vi "exampleloop.vi"() -> ()   [LabVIEW 2011]
uses:
  gumLV8p2/D/Labviewsoft/transport/GUMS/Kelvinox drivers/ITCAPPS - Copie.LLB/ITCSignal.ctl
  gumLV8p2/D/Labviewsoft/transport/GUMS/Kelvinox drivers/ITCAPPS - Copie.LLB/ITCSignals.ctl
  DAC/Visa name1.vi
  GlobalVar.vi
  stopButton.vi
  monochromatorcontrol/perHandlemonochromator.vi
  users/nicolas/PHySpec-SDK-1.0.0/Labview-example/libPhyspec/libPhyspec.lvlib
panel:
  out "Bloop gen":u32
  out "WVlenloop gen":u32
  out "Tloop gen":u32
  out "loopchange":u32
  out "DACindic":bool
  in  "Gain Cluster 2":T1={"Vsd"="Gate", "I 2probe 2"="Gate", "Vxy"="Gate", "Vxx"="Gate", "I leak BG"="Gate", "I leak TG"="Gate", "I Gain 1"=1000000.0, "V Gain 1"=1.0, "conversion factor BG"=1.0, "Vin / Vout 1"=1.0, "V Gain 2"=1.0, "Vin / Vout 2"=1.0, "V Gain 3"=1.0, "Vin / Vout 3"=1.0, "I Gain 2"=1000000.0, "I Gain 3"=1000000.0, "V BG"="Gate", "V TG"="Gate", "conversion factor TG"=1.0, "Vin / Vout 4"=1.0, "Vin / Vout 5"=1.0, "Manual Gain 1"=1.0, "Manual Gain 2"=1.0, "Manual Gain 3"=1.0} {"conversion factor TG" items=["1 V/V"=1.0, "4 V/V"=4.0, "15 V/V"=15.0, "30 V/V"=30.0, "45 V/V"=45.0]; "I Gain 3" items=["1"=1.0, "10"=10.0, "100"=100.0, "1K"=1000.0, "10K"=10000.0, "100K"=100000.0, "1M"=1000000.0, "10M"=10000000.0, "100M"=100000000.0, "1G"=1000000000.0]; "I Gain 2" items=["1"=1.0, "10"=10.0, "100"=100.0, "1K"=1000.0, "10K"=10000.0, "100K"=100000.0, "1M"=1000000.0, "10M"=10000000.0, "100M"=100000000.0, "1G"=1000000000.0]; "V Gain 3" items=["1"=1.0, "10"=10.0, "100"=100.0, "1K"=1000.0, "10K"=10000.0]; "V Gain 2" items=["1"=1.0, "10"=10.0, "100"=100.0, "1K"=1000.0, "10K"=10000.0]; "conversion factor BG" items=["1 V/V"=1.0, "4 V/V"=4.0, "15 V/V"=15.0, "30 V/V"=30.0, "45 V/V"=45.0]; "V Gain 1" items=["1"=1.0, "10"=10.0, "100"=100.0, "1K"=1000.0, "10K"=10000.0]; "I Gain 1" items=["1"=1.0, "10"=10.0, "100"=100.0, "1K"=1000.0, "10K"=10000.0, "100K"=100000.0, "1M"=1000000.0, "10M"=10000000.0, "100M"=100000000.0, "1G"=1000000000.0]}
  out "DAC 2 number":u8
  in  "EmptyAllArrays":bool
  in  "Sweep back to zero":bool
  out "counter":i32
  out "Num elements in col":i32[](array[numeric])
  out "Current col":i32
  in  "Refresh Rate [ms]":i32=1000 min=0
  out "Current sweep":dbl
  out "ITC ref":T2={"ITC"=0, "Signal"=enum."Sensor 3"}
  in  "Cancel run":bool
  out "DAC 1 number":u8
  out "DAC":refnum<visa-resource-name>
  out "K2400 2":refnum<visa-resource-name>
  out "Lockin1":refnum<visa-resource-name>
  out "K2400 1":refnum<visa-resource-name>
  out "Total sweep sequence":dbl[][](array[numeric])
  in  "Device Cluster":T4={"K2400 1"="", "K2400_1"=FALSE, "K2400 2"="", "K2400_2"=FALSE, "Lockin1"="", "Lockin1 present"=FALSE, "Lockin2"="", "Lockin2 present"=FALSE, "TIC"="", "Tcontrol"="OFF", "DMM1"="", "DMM1"=FALSE, "DMM2"="", "DMM2"=FALSE, "DAC"="", "DAC present"=FALSE, "DAC sweep"=0, "Bfield query"=FALSE, "Wvlen query"=FALSE, "ITC signal"={"ITC"=0, "Signal"=enum."Sensor 1"}, "DAC fix"=0}
  in  "Tab Control":T5(tab)
  in  "Sweep Toothsaw":bool
  in  "Loop Cluster":T6
  in  "START":bool
  in  "genTotalSequence":bool
  out "row state":i32[](array[numeric])
  out "Priority type array":string[](array[string])
  out "TotalPnts":dbl
  in  "Sweep back\nto zero?":bool
  in  "Conversion Factor Fix\n1 V = ??":dbl=1.0
  in  "Fix type":string(combo)
  in  "Sweep Bias":dbl[](array[numeric])
  in  "Fix Bias":dbl[](array[numeric])
  in  "Priority sweep":i32=2
  in  "Priority fix":i32=2
  in  "sweep start [V]":dbl=-1.0 min=-200.0 max=200.0
  in  "sweep stop [V]":dbl=-5.0 min=-250.0 max=250.0
  in  "Nb steps":i32=800
  in  "sweep stop 2 [V]":dbl min=-250.0 max=250.0
  in  "Nb steps 2":i32
  in  "Nb Sweep":i32=1
  in  "Nb steps fix2":i32
  in  "Fix stop 2":dbl min=-250.0 max=250.0
  in  "Nb steps fix":i32=800
  in  "Fix stop":dbl=-5.0 min=-250.0 max=250.0
  in  "Fix start":dbl=-1.0 min=-200.0 max=200.0
  in  "genSweepArray":bool
  in  "genFixArray":bool
  in  "Sweep Instrument":string(combo)
  in  "Conversion Factor Sweep\n1 V = ??":dbl=1.0
  in  "Fix Instrument":string(combo)
  in  "Sweep type":string(combo)
  in  "V step K2400 [V]":dbl=0.001
  in  "genSweepArray sweeploop":bool
  in  "genfixArray fixlooop simple":bool
  in  "T [K]":dbl[](array[numeric])
  in  "Priority T":i32=2
  in  "Nb T steps":i32=800
  in  "T stop [K]":dbl=-1.0 min=-200.0 max=200.0
  in  "T start [K]":dbl=-1.0 min=-200.0 max=200.0
  in  "genTarray":bool
  in  "Add T points":bool
  in  "Zero ramp Rate [T/min] 2":dbl=0.2 min=-200.0 max=200.0
  in  "Sweep Field back to zero":bool
  in  "B [T]":dbl[](array[numeric])
  in  "Priority B":i32=2
  in  "B start [T]":dbl=-1.0 min=-200.0 max=200.0
  in  "B stop [T]":dbl=-1.0 min=-200.0 max=200.0
  in  "Sweep Rate [T/min]":dbl=0.1 min=-200.0 max=200.0
  in  "Nb B steps":i32=800
  in  "GenBarray":bool
  in  "Add B points":bool
  in  "Set Persistent":bool=TRUE
  in  "Power stabilization":bool=TRUE
  in  "Wvlen Start [nm]":dbl=400.0
  in  "Wavelength [nm]":dbl[](array[numeric])
  in  "genWVLEN array":bool
  in  "Add wvlen points":bool
  in  "Nb Wvlen steps":i32=350
  in  "Wvlen stop [nm]":dbl=1100.0
  out "Laser Power [W]":dbl format="%#.2g"
  in  "File Basename":string
  out "Bias factor":dbl
  in  "SD bias [V]":dbl=-1.0 min=-200.0 max=200.0
  in  "Nb steps Increase 2":dbl=10.0
  in  "Gate Increase 2 (V)":dbl=0.1
  in  "Nb steps Increase":dbl=10.0
  in  "Gate Increase (V)":dbl=-0.1
  out "x .or. y?":bool
  in  "Step Delay (ms)":dbl=1000.0
  out "Total Progress":dbl(slide) scale=0.0..1.0
  in  "Nb Loop":i32
  out "Nb Loop Indicator":i32=2
  out "Nb Sweep Indicator":i32=3
  out "conversion factor sweep":dbl(ring)=1.0 items=["1 V/V"=1.0, "4 V/V"=4.0, "15 V/V"=15.0, "30 V/V"=30.0, "45 V/V"=45.0]
  in  "stop":bool
  in  "V step [V]":dbl=0.001
  in  "Folder Name":path=path "D:/users/marc/20180122_LiIon_EL/Freezing02/OutputHighT002p2.dat"
  # "Magnetic Field"
  # "Wavelength"
  # "IV Sweep Setting"
  # "IV Fix Setting"
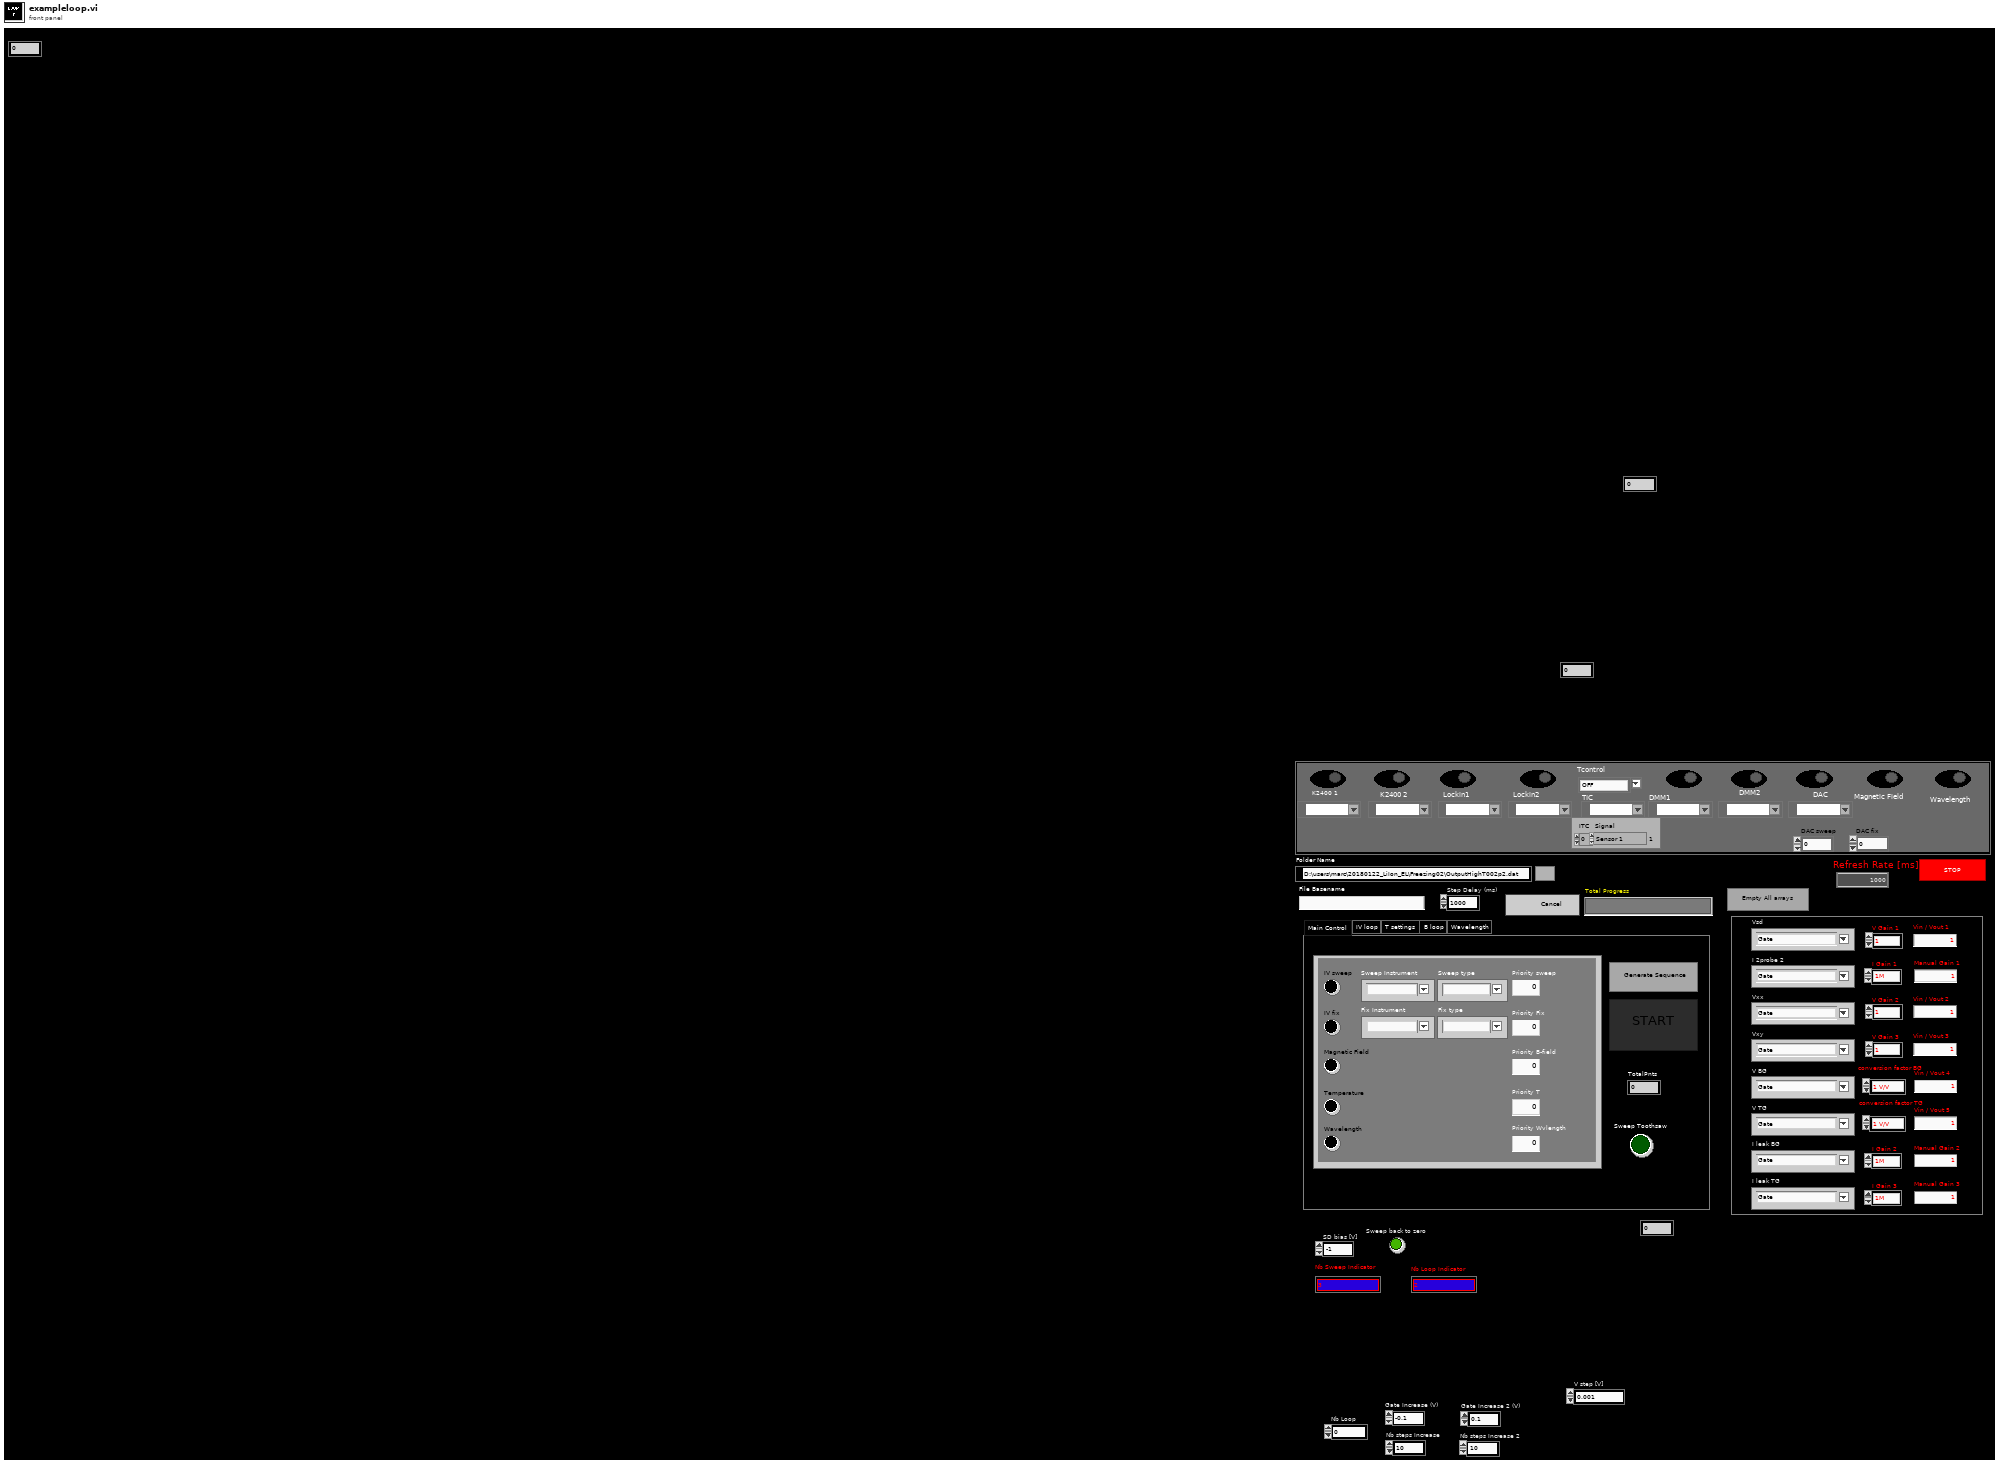
[diagram p1: front panel]
types:
  T1 = cluster{"Vsd":string, "I 2probe 2":string, "Vxy":string, "Vxx":string, "I leak BG":string, "I leak TG":string, "I Gain 1":dbl, "V Gain 1":dbl, "conversion factor BG":dbl, "Vin / Vout 1":dbl, "V Gain 2":dbl, "Vin / Vout 2":dbl, "V Gain 3":dbl, "Vin / Vout 3":dbl, "I Gain 2":dbl, "I Gain 3":dbl, "V BG":string, "V TG":string, "conversion factor TG":dbl, "Vin / Vout 4":dbl, "Vin / Vout 5":dbl, "Manual Gain 1":dbl, "Manual Gain 2":dbl, "Manual Gain 3":dbl}
  T2 = typedef "ITCSignal.ctl" = cluster{"ITC":u16, "Signal":T3}
  T3 = typedef "ITCSignals.ctl" = enum16{"Setpoint", "Sensor 1", "Sensor 2", "Sensor 3", "Needle Valve %", "Heater %"}
  T4 = cluster{"K2400 1":refnum<visa-resource-name>, "K2400_1":bool, "K2400 2":refnum<visa-resource-name>, "K2400_2":bool, "Lockin1":refnum<visa-resource-name>, "Lockin1 present":bool, "Lockin2":refnum<visa-resource-name>, "Lockin2 present":bool, "TIC":refnum<visa-resource-name>, "Tcontrol":string, "DMM1":refnum<visa-resource-name>, "DMM1":bool, "DMM2":refnum<visa-resource-name>, "DMM2":bool, "DAC":refnum<visa-resource-name>, "DAC present":bool, "DAC sweep":u8, "Bfield query":bool, "Wvlen query":bool, "ITC signal":T2, "DAC fix":u8}
  T5 = enum32{"Main Control", "IV loop", "T settings", "B loop", "Wavelength"}
  T6 = cluster{"Sweep Instrument":string, "Sweep type":string, "Fix Instrument":string, "Fix type":string, "IV sweep":bool, "IV fix":bool, "Magnetic Field":bool, "Temperature":bool, "Wavelength":bool, "Priority sweep":dbl, "Priority Fix":dbl, "Priority B-field":dbl, "Priority T":dbl, "Priority Wvlength":dbl}
  T7 = cluster{"Power Stabilization":bool, "Laser Power [W]":dbl, "Power precision":dbl}
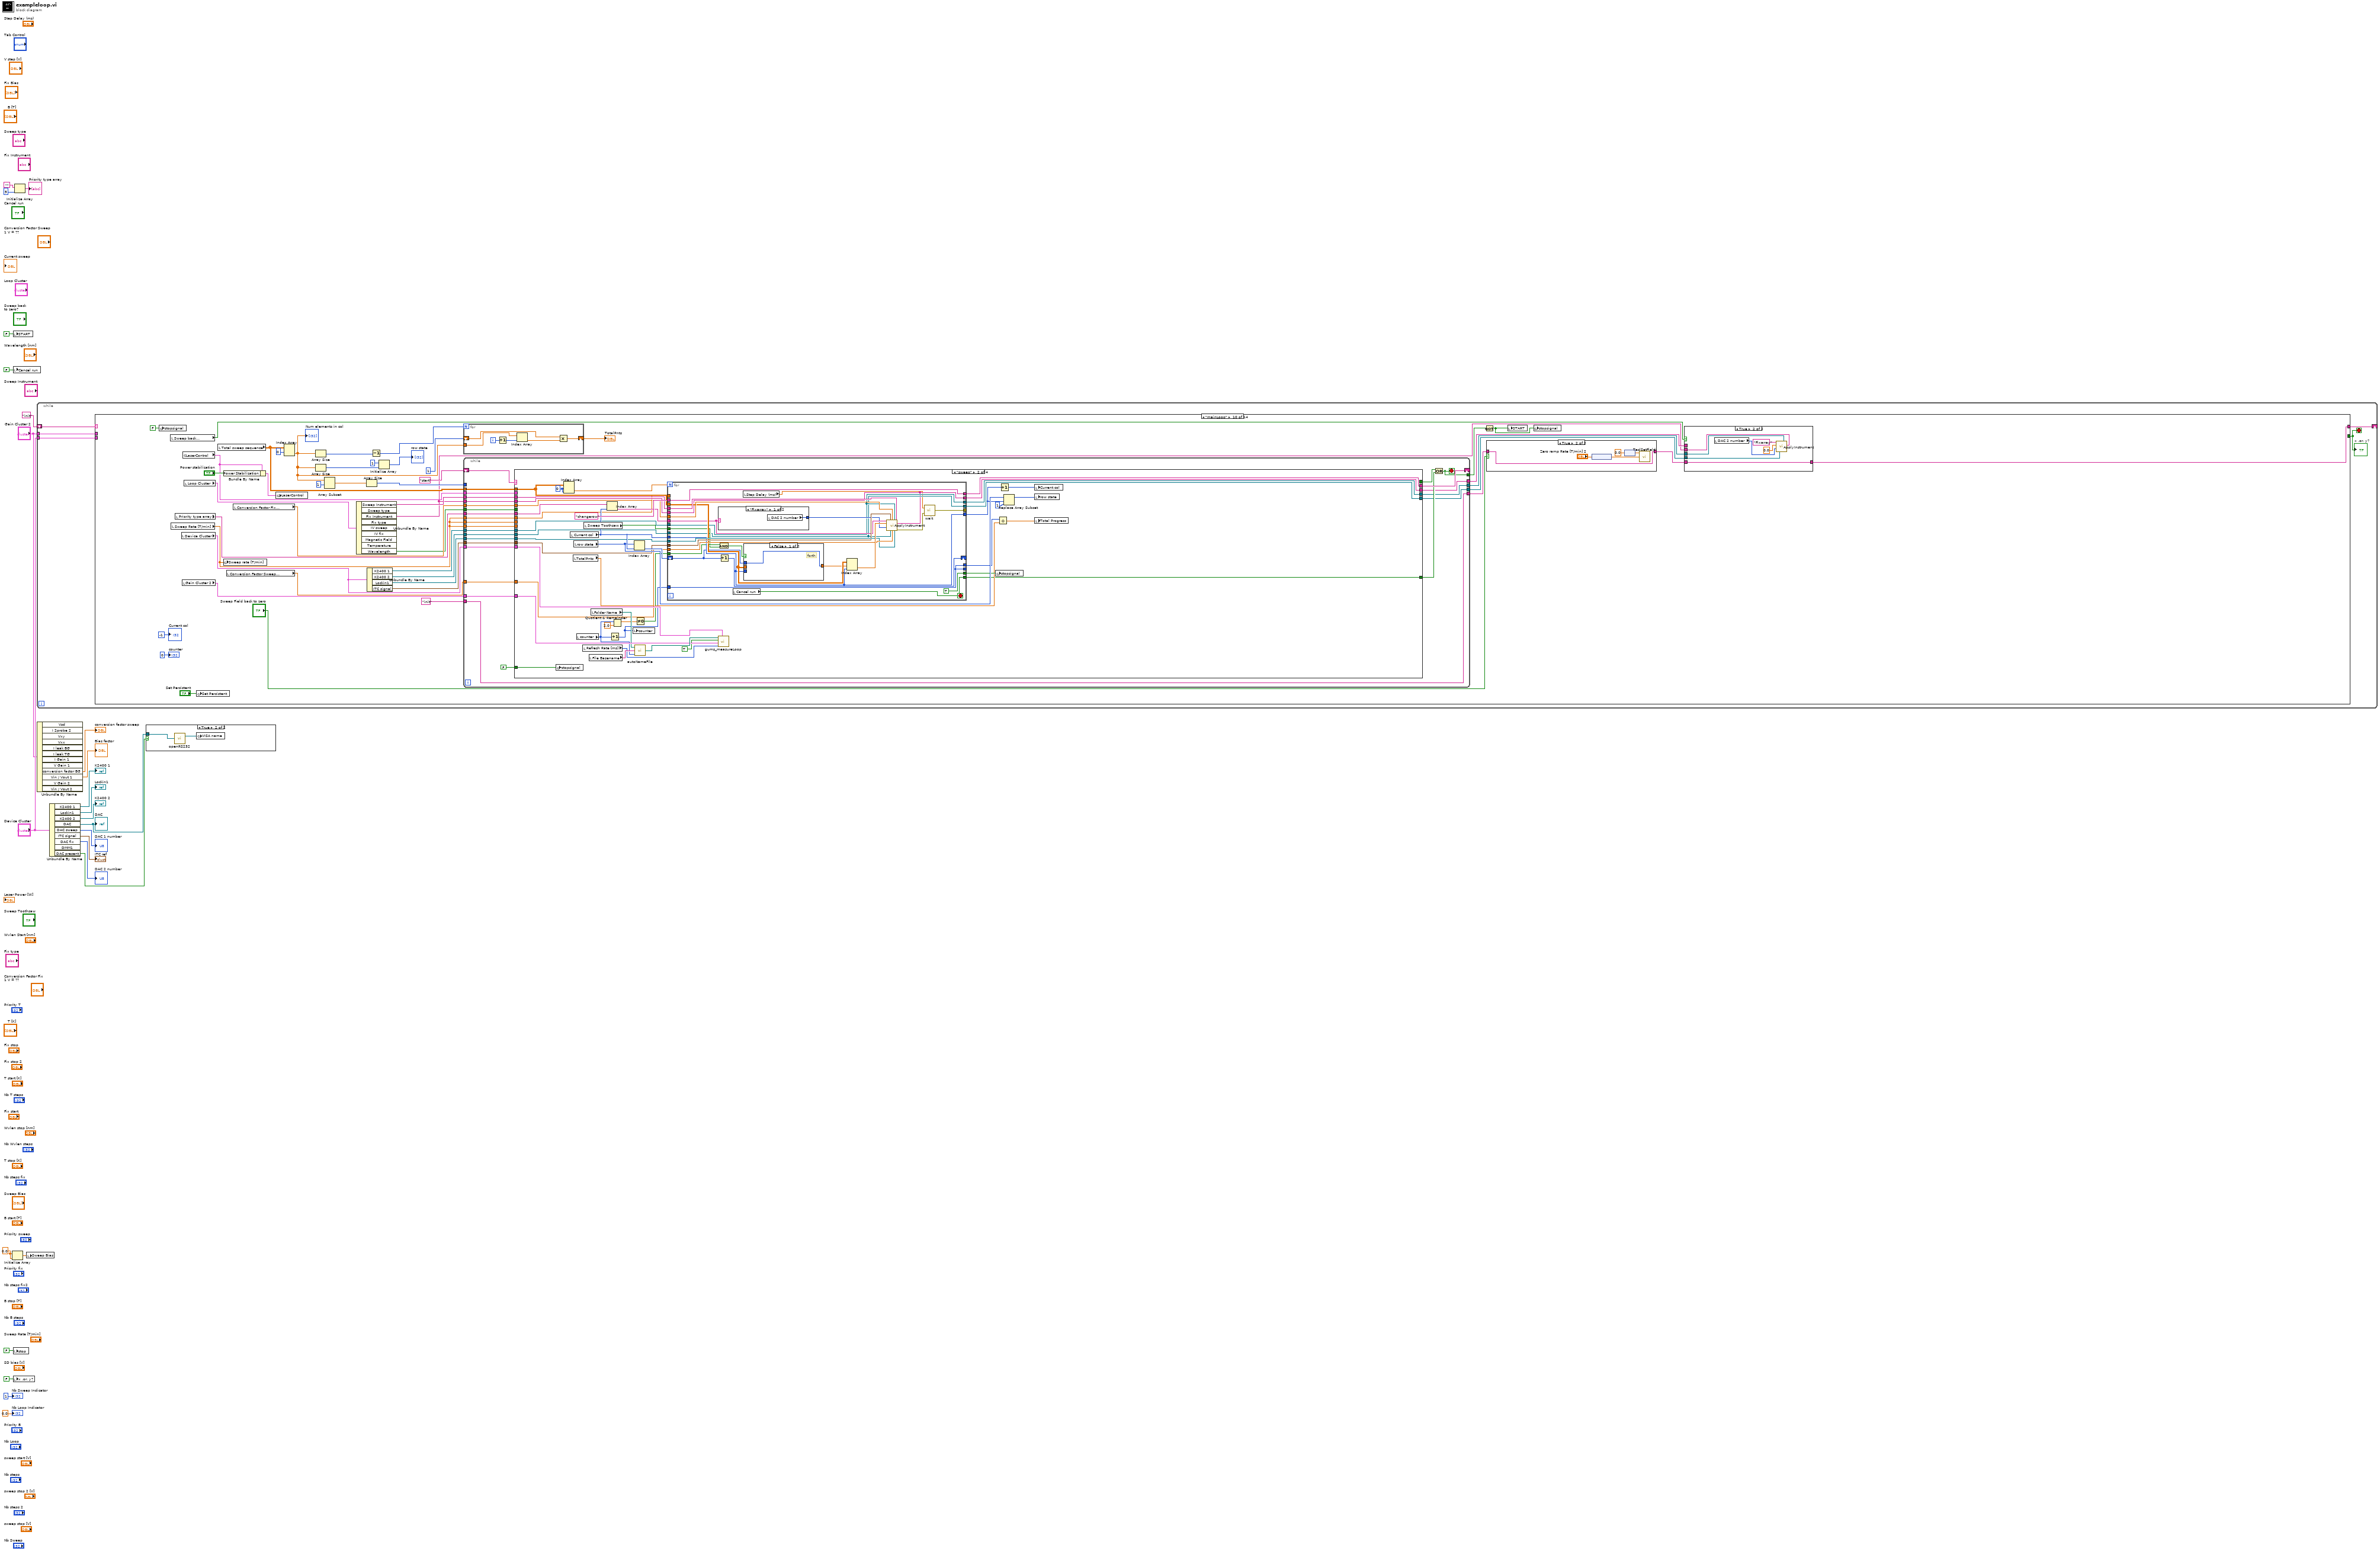
[diagram p0: block diagram]
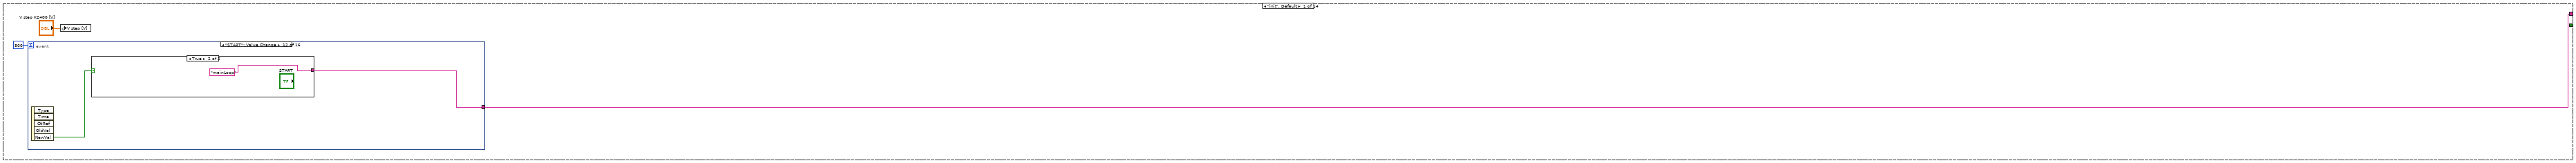
[diagram p3: hidden frame]
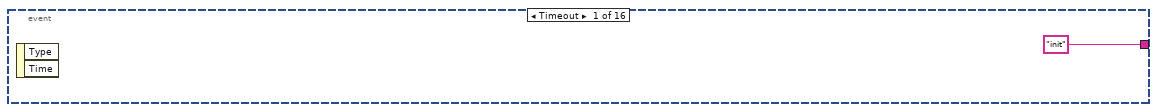
[diagram p4: hidden frame]
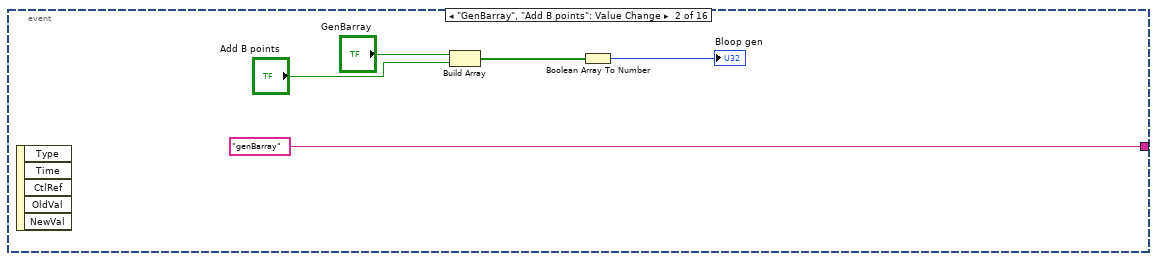
[diagram p5: hidden frame]
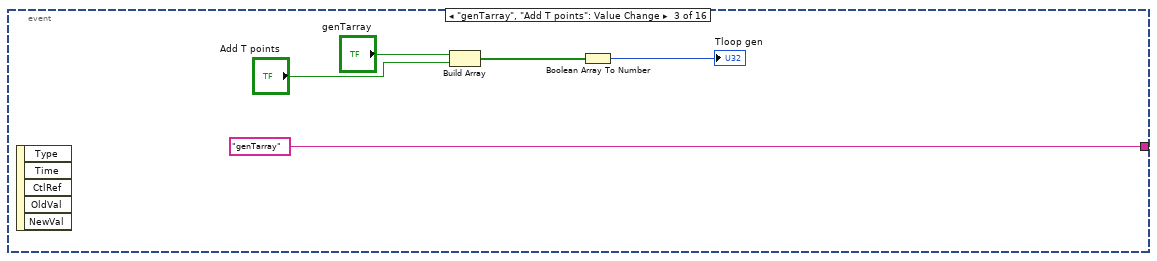
[diagram p6: hidden frame]
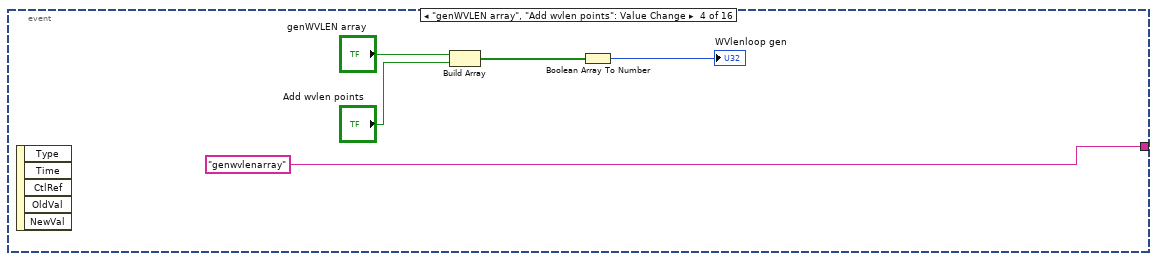
[diagram p7: hidden frame]
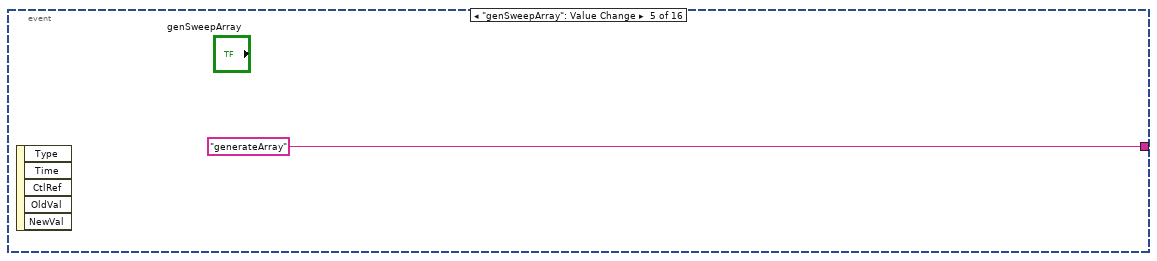
[diagram p8: hidden frame]
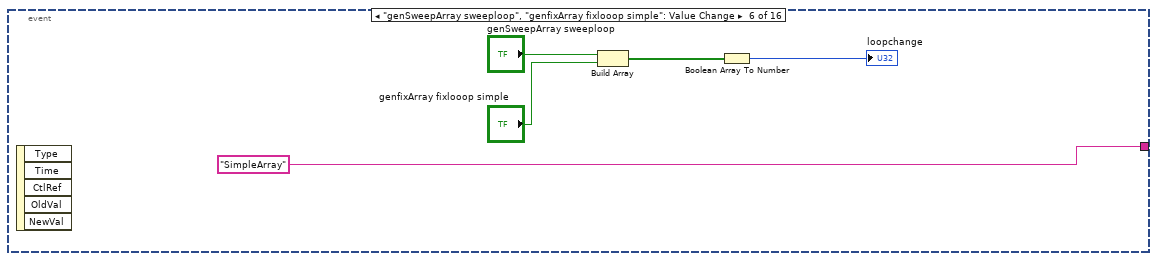
[diagram p9: hidden frame]
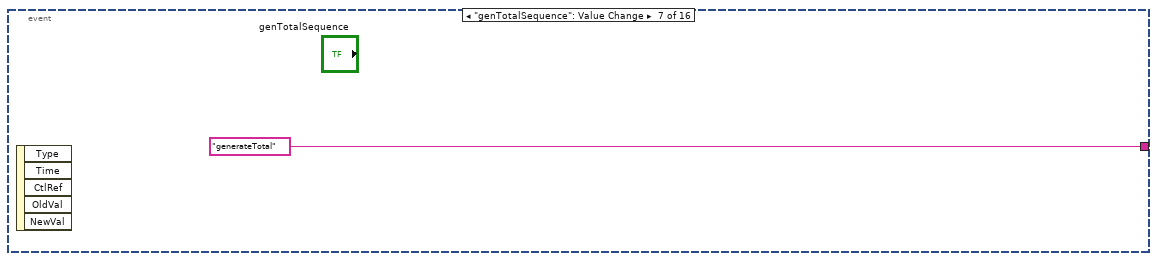
[diagram p10: hidden frame]
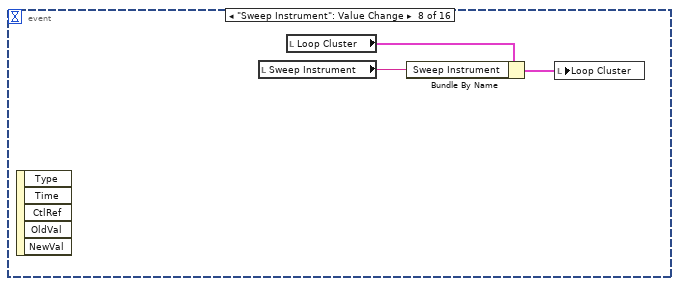
[diagram p11: hidden frame]
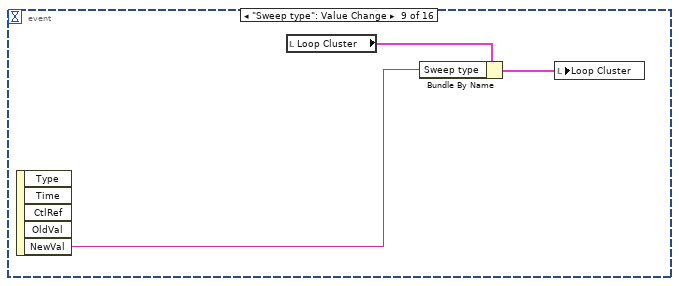
[diagram p12: hidden frame]
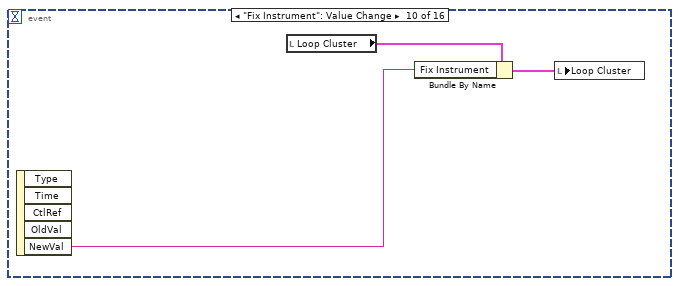
[diagram p13: hidden frame]
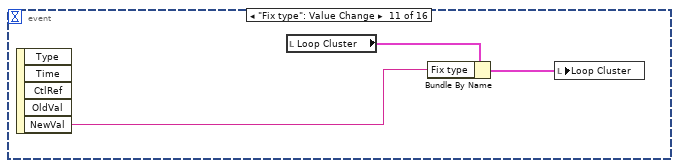
[diagram p14: hidden frame]
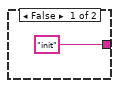
[diagram p15: hidden frame]
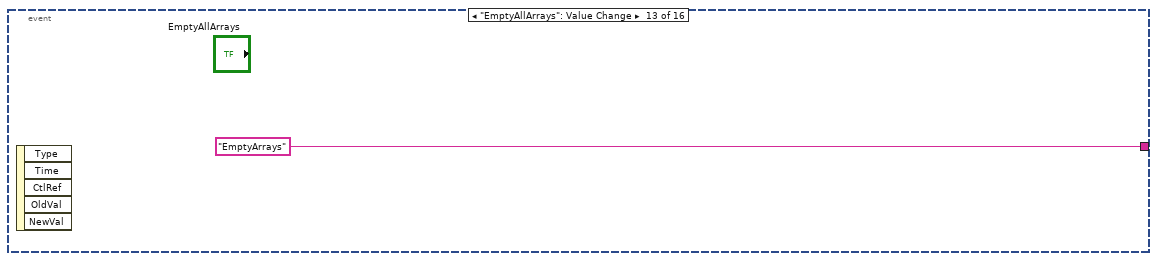
[diagram p16: hidden frame]
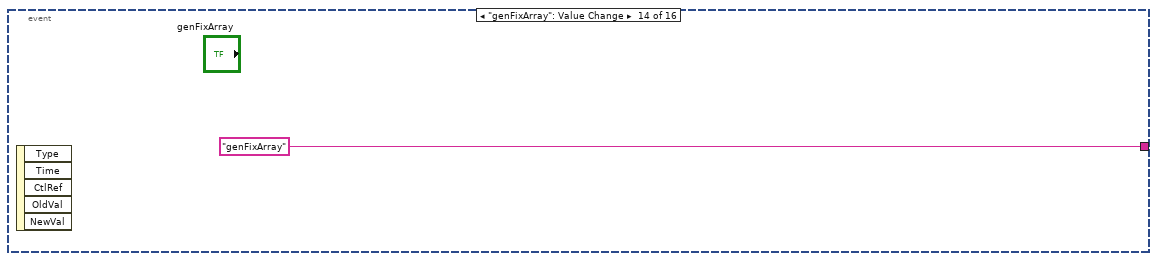
[diagram p17: hidden frame]
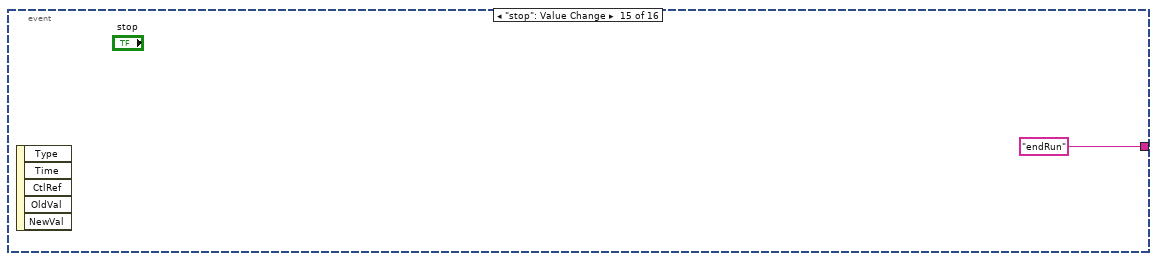
[diagram p18: hidden frame]
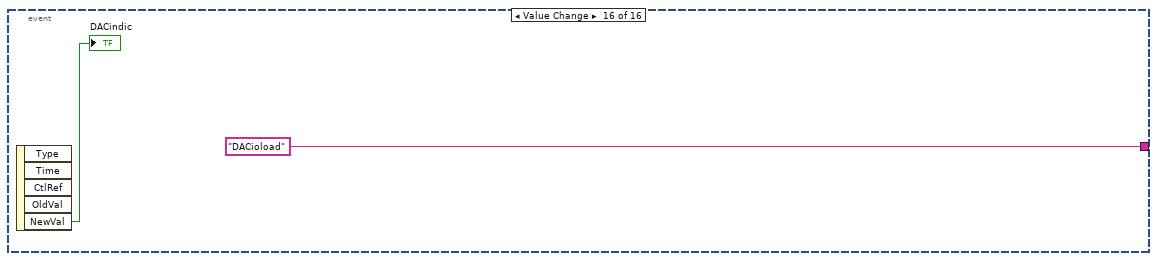
[diagram p19: hidden frame]
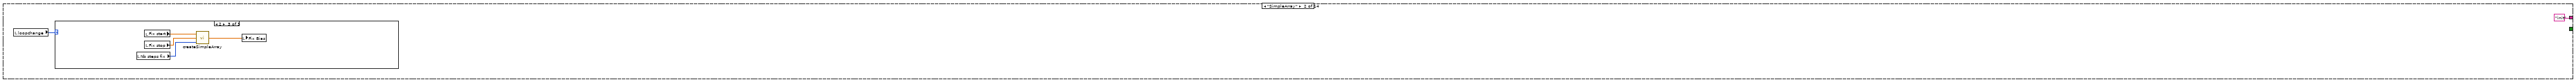
[diagram p20: hidden frame]
diagram:
  w6 = 0.0
  n1 = Initialize Array(w6, w6) -> (w7:dbl[])
  n2 = local write "START"(FALSE ("START")) -> ()
  n3 = local write "Cancel run"(FALSE ("Cancel run")) -> ()
  n4 = local write "stop"(FALSE ("stop")) -> ()
  n5 = local write "x .or. y?"(FALSE ("x .or. y?")) -> ()
  n6 = Initialize Array("", 5 ("dimension size")) -> (→"Priority type array":string[])
  n7 = local write "Sweep Bias"(w7) -> ()
  n8 = while {
    shift-right: [w25] -> _
    shift-left: "init" -> [w29]
    tunnel: "Gain Cluster 2" -> [w27]
    tunnel: "Device Cluster" -> [w26]
    stop <- w28 stop-if-true
    n9 = case shown="\"mainLoop\"" w29 {
      tunnel: [_ _ _ _ _ _ _ _ _ _ _ TRUE _ _] -> w28
      tunnel: [w31 "init" "init" "init" "init" "init" "init" "init" w248 w511 "generateArray" "" "init" w815] -> w25
      tunnel: w27 -> [_ _ _ _ _ _ _ _ _ _ _ _ _ _]
      tunnel: w26 -> [_ _ _ _ _ _ _ _ _ _ _ _ _ _]
      frame "init", Default {
        n10 = event shown="[11] \"START\": Value Change" {
          selector: _ -> [_ _ _ _ _ _ _ _ _ _ _ _ _ _ _ _]
          dyn-events: _ -> [_ _ _ _ _ _ _ _ _ _ _ _ _ _ _ _]
          timeout: 500 -> [_ _ _ _ _ _ _ _ _ _ _ _ _ _ _ _]
          tunnel: ["init" "genBarray" "genTarray" "genwvlenarray" "generateArray" "SimpleArray" "generateTotal" _ _ _ _ w68 "EmptyArrays" "genFixArray" "endRun" "DACioload"] -> w31
          event Timeout {
            n11 = event-data() -> ()  [unwired: 1 in, 2 out]
          }
          event "GenBarray", "Add B points": Value Change {
            n12 = event-data() -> ()  [unwired: 1 in, 5 out]
            n13 = Build Array("GenBarray", "Add B points") -> (w37:bool[])
            n14 = Boolean Array To Number(Boolean array=w37) -> (number=→"Bloop gen":u32)
          }
          event "genTarray", "Add T points": Value Change {
            n15 = event-data() -> ()  [unwired: 1 in, 5 out]
            n16 = Build Array("genTarray", "Add T points") -> (w42:bool[])
            n17 = Boolean Array To Number(Boolean array=w42) -> (number=→"Tloop gen":u32)
          }
          event "genWVLEN array", "Add wvlen points": Value Change {
            n18 = event-data() -> ()  [unwired: 1 in, 5 out]
            n19 = Build Array("genWVLEN array", "Add wvlen points") -> (w47:bool[])
            n20 = Boolean Array To Number(Boolean array=w47) -> (number=→"WVlenloop gen":u32)
          }
          event "genSweepArray": Value Change {
            n21 = event-data() -> ()  [unwired: 1 in, 5 out]
          }
          event "genSweepArray sweeploop", "genfixArray fixlooop simple": Value Change {
            n22 = event-data() -> ()  [unwired: 1 in, 5 out]
            n23 = Build Array("genSweepArray sweeploop", "genfixArray fixlooop simple") -> (w51:bool[])
            n24 = Boolean Array To Number(Boolean array=w51) -> (number=→"loopchange":u32)
          }
          event "genTotalSequence": Value Change {
            n25 = event-data() -> ()  [unwired: 1 in, 5 out]
          }
          event "Sweep Instrument": Value Change {
            n26 = event-data() -> ()  [unwired: 1 in, 5 out]
            n27 = local read "Sweep Instrument"() -> (w57:string)
            n28 = local read "Loop Cluster"() -> (w58:T6)
            n29 = Bundle By Name(cluster=w58, "Sweep Instrument"=w57) -> (w56:T6)
            n30 = local write "Loop Cluster"(w56) -> ()
          }
          event "Sweep type": Value Change {
            n31 = event-data() -> ("NewVal"=w59:string)  [unwired: 1 in, 4 out]
            n32 = local read "Loop Cluster"() -> (w61:T6)
            n33 = Bundle By Name(cluster=w61, "Sweep type"=w59) -> (w60:T6)
            n34 = local write "Loop Cluster"(w60) -> ()
          }
          event "Fix Instrument": Value Change {
            n35 = event-data() -> ("NewVal"=w62:string)  [unwired: 1 in, 4 out]
            n36 = local read "Loop Cluster"() -> (w63:T6)
            n37 = Bundle By Name(cluster=w63, "Fix Instrument"=w62) -> (w64:T6)
            n38 = local write "Loop Cluster"(w64) -> ()
          }
          event "Fix type": Value Change {
            n39 = event-data() -> ("NewVal"=w67:string)  [unwired: 1 in, 4 out]
            n40 = local read "Loop Cluster"() -> (w66:T6)
            n41 = Bundle By Name(cluster=w66, "Fix type"=w67) -> (w65:T6)
            n42 = local write "Loop Cluster"(w65) -> ()
          }
          event "START": Value Change {
            n43 = event-data() -> ("NewVal"=w69:bool)  [unwired: 1 in, 4 out]
            n44 = case shown="True" w69 {
              tunnel: ["init" "mainLoop"] -> w68
              frame False {
              }
              frame True {
              }
            }
          }
          event "EmptyAllArrays": Value Change {
            n45 = event-data() -> ()  [unwired: 1 in, 5 out]
          }
          event "genFixArray": Value Change {
            n46 = event-data() -> ()  [unwired: 1 in, 5 out]
          }
          event "stop": Value Change {
            n47 = event-data() -> ()  [unwired: 1 in, 5 out]
          }
          event "Device Cluster.DAC present": Value Change {
            n48 = event-data() -> ("NewVal"=→"DACindic":bool)  [unwired: 1 in, 4 out]
          }
        }
        n49 = global write "GlobalVar.vi" "V step [V]"("V step K2400 [V]") -> ()
      }
      frame "SimpleArray" {
        n50 = local read "loopchange"() -> (w77:u32)
        n51 = case shown="2" w77 {
          frame 0, Default {
          }
          frame 1 {
            n52 = local read "Nb steps"() -> (w81:i32)
            n53 = local read "sweep start [V]"() -> (w79:dbl)
            n54 = local read "sweep stop [V]"() -> (w80:dbl)
            n55 = call "createSimpleArray.vi"("nbpoint1"=w81, "Bgstop"=w80, "Bgstart"=w79) -> ("Outarray"=w82:dbl[])
            n56 = local write "Sweep Bias"(w82) -> ()
          }
          frame 2 {
            n57 = local read "Nb steps fix"() -> (w83:i32)
            n58 = local read "Fix start"() -> (w85:dbl)
            n59 = local read "Fix stop"() -> (w84:dbl)
            n60 = call "createSimpleArray.vi"("nbpoint1"=w83, "Bgstop"=w84, "Bgstart"=w85) -> ("Outarray"=w86:dbl[])
            n61 = local write "Fix Bias"(w86) -> ()
          }
        }
      }
      frame "generateTotal" {
        n62 = local read "Loop Cluster"() -> (w95:T6)
        n63 = Unbundle By Name(w95) -> ("IV sweep"=w115:bool, "IV fix"=w114:bool, "Magnetic Field"=w113:bool, "Temperature"=w112:bool, "Wavelength"=w111:bool, "Priority sweep"=w106:dbl, "Priority Fix"=w105:dbl, "Priority B-field"=w104:dbl, "Priority T"=w103:dbl, "Priority Wvlength"=w98:dbl)
        n64 = Build Array(w115, w114, w113, w112, w111) -> (w109:bool[])
        n65 = Decrement(x=w106) -> (x-1=w99:dbl)
        n66 = Decrement(x=w105) -> (x-1=w100:dbl)
        n67 = Decrement(x=w104) -> (x-1=w101:dbl)
        n68 = Decrement(x=w103) -> (x-1=w102:dbl)
        n69 = Decrement(x=w98) -> (x-1=w97:dbl)
        n70 = Boolean To (0,1)(Boolean=w109) -> (0, 1=w110:i16[])
        n71 = Add Array Elements(numeric array=w110) -> (sum=w108:i16)
        n72 = for {
          N: w108 -> [_]
          shift-right: [w140] -> w90
          shift-left: dbl[][] [] ("Array In") -> [w141]
          tunnel: w102 -> [w137]
          tunnel: w101 -> [w138]
          tunnel: w100 -> [w139]
          tunnel: w99 -> [w131]
          tunnel: w97 -> [w133]
          shift-right: [w126] -> w94
          shift-left: string[] [] -> [w124]
          i -> [w134]
          n73 = Equal?(x=w131, y=w134) -> (x = y?=w130:bool)
          n74 = Equal?(x=w139, y=w134) -> (x = y?=w129:bool)
          n75 = Equal?(x=w138, y=w134) -> (x = y?=w128:bool)
          n76 = Equal?(x=w137, y=w134) -> (x = y?=w127:bool)
          n77 = Equal?(x=w133, y=w134) -> (x = y?=w132:bool)
          n78 = Build Array(w130, w129, w128, w127, w132) -> (w136:bool[])
          n79 = Boolean Array To Number(Boolean array=w136) -> (number=w135:u32)
          n80 = case shown="16" w135 {
            tunnel: [_ "sweeparray" "Fixarray" "Bfield" ("Fix Instrument") "Temperature" "wavelength"] -> w125
            tunnel: [_ w143 w145 w146 w148 w150] -> w123
            frame 0, Default {
            }
            frame 1 {
              n81 = local read "Sweep Bias"() -> (w143:dbl[])
            }
            frame 2 {
              n82 = local read "Fix Bias"() -> (w145:dbl[])
            }
            frame 4 {
              n83 = local read "B [T]"() -> (w146:dbl[])
            }
            frame 8 {
              n84 = local read "T [K]"() -> (w148:dbl[])
            }
            frame 16 {
              n85 = local read "Wavelength [nm]"() -> (w150:dbl[])
            }
          }
          n86 = call "generateFinalArray.vi"("new array"=w123, "Array In"=w141) -> ("Array out"=w140:dbl[][])
          n87 = Build Array (concatenate)(w124, w125) -> (w126:string[])
        }
        "Total sweep sequence" <- w90
        n88 = local write "Priority type array"(w94) -> ()
        n89 = Index Array(array=w90, index (row)=0) -> (element=w87:dbl[])  [unwired: 1 in]
        n90 = Array Size(array=w87) -> (size(s)=w89:i32)
        n91 = Decrement(x=w89) -> (x-1=w88:i32)
        n92 = for {
          N: w88 -> [_]
          tunnel: w87 -> [w120]
          shift-right: [w117] -> w93
          shift-left: 1 ("index") -> [w118]
          i -> [w122]
          n93 = Increment(x=w122) -> (x+1=w121:i32)
          n94 = Index Array(array=w120, index=w121) -> (element=w119:dbl)
          n95 = Multiply(x=w118, y=w119) -> (x*y=w117:dbl)
        }
        n96 = local write "TotalPnts"(w93) -> ()
      }
      frame "generateArray" {
        w153 = 0.0 ("element")
        n97 = local read "Nb Sweep"() -> (w160:i32)
        n98 = local read "Priority type array"() -> (w158:string[])
        n99 = local read "Priority sweep"() -> (w154:i32)
        n100 = Initialize Array(w153, w153) -> (w152:dbl[])
        n101 = for {
          N: w160 -> [_]
          shift-right: [w164] -> w159
          shift-left: w152 -> [w163]
          n102 = local read "Nb steps 2"() -> (w168:i32)
          n103 = local read "Nb steps"() -> (w169:i32)
          n104 = local read "sweep stop 2 [V]"() -> (w166:dbl)
          n105 = local read "sweep start [V]"() -> (w167:dbl)
          n106 = local read "sweep stop [V]"() -> (w165:dbl)
          n107 = call "createLoopArray.vi"("Bgstop"=w165, "Bgstop2"=w166, "nbpoint1"=w169, "nbpoint2"=w168, "Bgstart"=w167) -> ("Outarray"=w162:dbl[])
          n108 = Build Array (concatenate)(w163, w162) -> (w164:dbl[])
        }
        n109 = Decrement(x=w154) -> (x-1=w155:i32)
        n110 = Replace Array Subset(array=w158, new element="sweeparray" ("new element/subarray"), index=w155) -> (w157:string[])
        n111 = local write "Priority type array"(w157) -> ()
        n112 = local write "Sweep Bias"(w159) -> ()
      }
      frame "genFixArray" {
        n113 = local read "Priority fix"() -> (w170:i32)
        n114 = local read "Nb Sweep"() -> (w177:i32)
        n115 = local read "Fix Bias"() -> (w176:dbl[])
        n116 = local read "Priority type array"() -> (w174:string[])
        n117 = for {
          N: w177 -> [_]
          shift-right: [w181] -> w175
          shift-left: w176 -> [w180]
          n118 = local read "Nb steps fix"() -> (w186:i32)
          n119 = local read "Fix stop 2"() -> (w183:dbl)
          n120 = local read "Fix start"() -> (w184:dbl)
          n121 = local read "Fix stop"() -> (w182:dbl)
          n122 = local read "Nb steps fix2"() -> (w185:i32)
          n123 = call "createLoopArray.vi"("Bgstop"=w182, "Bgstop2"=w183, "nbpoint1"=w186, "nbpoint2"=w185, "Bgstart"=w184) -> ("Outarray"=w179:dbl[])
          n124 = Build Array (concatenate)(w180, w179) -> (w181:dbl[])
        }
        n125 = Decrement(x=w170) -> (x-1=w171:i32)
        n126 = Replace Array Subset(array=w174, new element="Fixarray" ("new element/subarray"), index=w171) -> (w173:string[])
        n127 = local write "Priority type array"(w173) -> ()
        n128 = local write "Fix Bias"(w175) -> ()
      }
      frame "genTarray" {
        n129 = local read "Nb T steps"() -> (w189:i32)
        n130 = local read "Tloop gen"() -> (w192:u32)
        n131 = local read "T start [K]"() -> (w191:dbl)
        n132 = local read "T stop [K]"() -> (w190:dbl)
        n133 = local read "T [K]"() -> (w188:dbl[])
        n134 = case shown="2" w192 {
          tunnel: w191 -> [_ w198 w204]
          tunnel: w190 -> [_ w197 w203]
          tunnel: w189 -> [_ w196 w202]
          tunnel: [w194 w195 w199] -> w187
          tunnel: w188 -> [w194 _ w201]
          frame 0, Default {
          }
          frame 1 {
            n135 = call "createSimpleArray.vi"("nbpoint1"=w196, "Bgstop"=w197, "Bgstart"=w198) -> ("Outarray"=w195:dbl[])
          }
          frame 2 {
            n136 = call "createSimpleArray.vi"("nbpoint1"=w202, "Bgstop"=w203, "Bgstart"=w204) -> ("Outarray"=w200:dbl[])
            n137 = Insert Into Array(array=w201, new element=w200) -> (w199:dbl[])  [unwired: 1 in]
          }
        }
        n138 = local write "T [K]"(w187) -> ()
      }
      frame "genBarray" {
        n139 = local read "Nb B steps"() -> (w207:i32)
        n140 = local read "Bloop gen"() -> (w210:u32)
        n141 = local read "B start [T]"() -> (w209:dbl)
        n142 = local read "B stop [T]"() -> (w208:dbl)
        n143 = local read "B [T]"() -> (w206:dbl[])
        n144 = case shown="2" w210 {
          tunnel: w209 -> [_ w216 w222]
          tunnel: w208 -> [_ w215 w221]
          tunnel: w207 -> [_ w214 w220]
          tunnel: [w212 w213 w217] -> w205
          tunnel: w206 -> [w212 _ w219]
          frame 0, Default {
          }
          frame 1 {
            n145 = call "createSimpleArray.vi"("nbpoint1"=w214, "Bgstop"=w215, "Bgstart"=w216) -> ("Outarray"=w213:dbl[])
          }
          frame 2 {
            n146 = call "createSimpleArray.vi"("nbpoint1"=w220, "Bgstop"=w221, "Bgstart"=w222) -> ("Outarray"=w218:dbl[])
            n147 = Insert Into Array(array=w219, new element=w218) -> (w217:dbl[])  [unwired: 1 in]
          }
        }
        n148 = local write "B [T]"(w205) -> ()
      }
      frame "genwvlenarray" {
        n149 = local read "Wavelength [nm]"() -> (w224:dbl[])
        n150 = local read "Wvlen Start [nm]"() -> (w227:dbl)
        n151 = local read "Wvlen stop [nm]"() -> (w226:dbl)
        n152 = local read "Nb Wvlen steps"() -> (w225:i32)
        n153 = local read "WVlenloop gen"() -> (w228:u32)
        n154 = case shown="2" w228 {
          tunnel: w227 -> [_ w234 w240]
          tunnel: w226 -> [_ w233 w239]
          tunnel: w225 -> [_ w232 w238]
          tunnel: [w230 w231 w235] -> w223
          tunnel: w224 -> [w230 _ w237]
          frame 0, Default {
          }
          frame 1 {
            n155 = call "createSimpleArray.vi"("nbpoint1"=w232, "Bgstop"=w233, "Bgstart"=w234) -> ("Outarray"=w231:dbl[])
          }
          frame 2 {
            n156 = call "createSimpleArray.vi"("nbpoint1"=w238, "Bgstop"=w239, "Bgstart"=w240) -> ("Outarray"=w236:dbl[])
            n157 = Insert Into Array(array=w237, new element=w236) -> (w235:dbl[])  [unwired: 1 in]
          }
        }
        n158 = local write "Wavelength [nm]"(w223) -> ()
      }
      frame "_mainLoop_old" {
        w262 = 0 ("index (row)")
        n159 = global write "stopButton.vi" "stopsignal"(FALSE ("stopsignal")) -> ()
        n160 = local read "Priority type array"() -> (w257:string[])
        n161 = local read "Total sweep sequence"() -> (w258:dbl[][])
        n162 = Index Array(array=w258, index (row)=w262, index (col)=3 ("index (row)")) -> (element=w246:dbl)
        n163 = Index Array(array=w258, index (row)=w262, index (col)=2 ("index (row)")) -> (element=w245:dbl)
        n164 = Index Array(array=w258, index (row)=w262, index (col)=1 ("index (row)")) -> (element=w244:dbl)
        n165 = Index Array(array=w258, index (row)=w262, index (col)=0 ("index (row)")) -> (element=w243:dbl)
        n166 = Compound Arithmetic op=MULTIPLY(w246, w245, w244, w243) -> (w242:dbl)
        n167 = Index Array(array=w257, index=0 ("index (row)")) -> (element=w249:string)
        n168 = Index Array(array=w257, index=2 ("index (row)")) -> (element=w250:string)
        n169 = Index Array(array=w257, index=1 ("index (row)")) -> (element=w251:string)
        n170 = Index Array(array=w257, index=3 ("index (row)")) -> (element=w252:string)
        n171 = for {
          N: w246 -> [w270]
          tunnel: w245 -> [w283]
          tunnel: w244 -> [w282]
          tunnel: w243 -> [w281]
          tunnel: w258 -> [w279]
          tunnel: w252 -> [w277]
          tunnel: w251 -> [w276]
          tunnel: w250 -> [w275]
          tunnel: w249 -> [w274]
          tunnel: [w272] -> w248
          tunnel: "init" -> [w272]
          tunnel: w242 -> [w267]
          tunnel: [FALSE] -> w241
          i -> [w269]
          stop <- w266 stop-if-true
          n172 = Multiply(x=w270, y=w269) -> (x*y=w268:i32)
          n173 = Increment(x=w269) -> (x+1=w271:i32)
          n174 = Index Array(array=w279, index (row)=w271, index (col)=3 ("disabled index (col)")) -> (element=w278:dbl)
          n175 = case shown="\"Bfield\"" w277 {
            selector: w277 -> [w284 _ _ _ _]
            tunnel: w278 -> [w287 w301 _ w318 _]
            tunnel: [w284 _ _ _ _] -> w273
            frame "sweeparray" {
              n176 = local read "Sweep Instrument"() -> (w285:string)
              n177 = local read "Conversion Factor Sweep\n1 V = ??"() -> (w288:dbl)
              n178 = Divide(x=w287, y=w288) -> (x/y=w286:dbl)
              n179 = case shown="\"Lockin\"" w285 {
                tunnel: w286 -> [_ w289 w292 w293 w295]
                frame Default {
                }
                frame "DAC" {
                  n180 = Multiply(x=w289, y=1000.0) -> (x*y=w291:dbl)
                  n181 = call "DAC set.vi"("DAC set [mV]"=w291) -> ()  [unwired: 2 in, 1 out]
                }
                frame "K2400_2" {
                  n182 = call "K2400_ApplyVOLTsafe_GUMS.vi"("Voltage target [V]"=w292) -> ()  [unwired: 1 in, 1 out]
                }
                frame "K2400_1" {
                  n183 = call "K2400_ApplyVOLTsafe_GUMS.vi"("Voltage target [V]"=w293) -> ()  [unwired: 1 in, 1 out]
                }
                frame "Lockin" {
                  n184 = Number To Fractional String(number=w295) -> (F-format string=w298:string)  [unwired: 3 out]
                  n185 = local read "Lockin1"() -> (w294:refnum<visa-resource-name>)
                  n186 = Concatenate Strings("SLVL " ("chaîne"), w298) -> (w296:string)
                  n187 = VISA Write(VISA resource name=w294, write buffer=w296) -> ()  [unwired: 1 in, 3 out]
                }
              }
            }
            frame "Fixarray" {
              n188 = local read "Fix Instrument"() -> (w299:string)
              n189 = local read "Conversion Factor Fix\n1 V = ??"() -> (w302:dbl)
              n190 = Divide(x=w301, y=w302) -> (x/y=w300:dbl)
              n191 = case shown="\"K2400_1\"" w299 {
                tunnel: w300 -> [_ w305 w309 w311 w313]
                frame Default {
                }
                frame "DAC" {
                  n192 = Multiply(x=w305, y=1000.0) -> (x*y=w307:dbl)
                  n193 = local read "DAC 1 number"() -> (w303:u8)
                  n194 = local read "DAC"() -> (w304:refnum<visa-resource-name>)
                  n195 = call "DAC set.vi"("DAC number"=w303, "DAC set [mV]"=w307, "DAC COM port"=w304) -> ()  [unwired: 1 out]
                }
                frame "K2400_2" {
                  n196 = local read "K2400 2"() -> (w308:refnum<visa-resource-name>)
                  n197 = call "K2400_ApplyVOLTsafe_GUMS.vi"("Voltage target [V]"=w309, "VISA Resource Name"=w308) -> ()  [unwired: 1 out]
                }
                frame "K2400_1" {
                  n198 = local read "K2400 1"() -> (w310:refnum<visa-resource-name>)
                  n199 = call "K2400_ApplyVOLTsafe_GUMS.vi"("Voltage target [V]"=w311, "VISA Resource Name"=w310) -> ()  [unwired: 1 out]
                }
                frame "Lockin" {
                  n200 = Number To Fractional String(number=w313) -> (F-format string=w316:string)  [unwired: 3 out]
                  n201 = local read "Lockin1"() -> (w312:refnum<visa-resource-name>)
                  n202 = Concatenate Strings("SLVL " ("chaîne"), w316) -> (w314:string)
                  n203 = VISA Write(VISA resource name=w312, write buffer=w314) -> ()  [unwired: 1 in, 3 out]
                }
              }
            }
            frame Default {
            }
            frame "Bfield" {
              n204 = node(w318) -> (w317:dbl[unit])
              n205 = local read "Sweep Rate [T/min]"() -> (w319:dbl)
              n206 = node(w319) -> (w320:dbl[unit])
              n207 = call "TeslSetField.vi"("Sweep rate"=w320, "Field required:"=w317) -> ()  [unwired: 2 in, 2 out]
            }
            frame "Temperature" {
              n208 = local read "ITC ref"() -> (w321:T2)
              n209 = call "Tloop.vi"("ITCSignal"=w321, "Regulate ?"=TRUE) -> ()  [unwired: 3 in, 2 out]
            }
          }
          n210 = for {
            N: w283 -> [w329]
            tunnel: w282 -> [w340]
            tunnel: w281 -> [w339]
            tunnel: w279 -> [w338]
            tunnel: w276 -> [w335]
            tunnel: w275 -> [w334]
            tunnel: w274 -> [w333]
            tunnel: w273 -> [_]
            tunnel: w268 -> [w330]
            tunnel: w267 -> [w324]
            tunnel: [w323] -> w266
            i -> [w328]
            stop <- w323 stop-if-true
            n211 = Multiply(x=w329, y=w330) -> (x*y=w326:i32)
            n212 = Multiply(x=w329, y=w328) -> (x*y=w327:i32)
            n213 = Increment(x=w328) -> (x+1=w331:i32)
            n214 = Add(x=w327, y=w326) -> (x+y=w325:i32)
            n215 = Index Array(array=w338, index (row)=w331, index (col)=2 ("disabled index (col)")) -> (element=w336:dbl)
            n216 = case shown="\"Bfield\"" w335 {
              selector: w335 -> [_ w352 _ _ _]
              tunnel: w336 -> [w343 w355 _ w370 _]
              tunnel: [_ w352 _ _ _] -> w332
              frame "sweeparray" {
                n217 = local read "Sweep Instrument"() -> (w341:string)
                n218 = local read "Conversion Factor Sweep\n1 V = ??"() -> (w344:dbl)
                n219 = Divide(x=w343, y=w344) -> (x/y=w342:dbl)
                n220 = case shown="\"DAC\"" w341 {
                  tunnel: w342 -> [_ _ w345 w346 w348]
                  frame Default {
                  }
                  frame "DAC" {
                  }
                  frame "K2400_2" {
                    n221 = call "K2400_ApplyVOLTsafe_GUMS.vi"("Voltage target [V]"=w345) -> ()  [unwired: 1 in, 1 out]
                  }
                  frame "K2400_1" {
                    n222 = call "K2400_ApplyVOLTsafe_GUMS.vi"("Voltage target [V]"=w346) -> ()  [unwired: 1 in, 1 out]
                  }
                  frame "Lockin" {
                    n223 = Number To Fractional String(number=w348) -> (F-format string=w351:string)  [unwired: 3 out]
                    n224 = local read "Lockin1"() -> (w347:refnum<visa-resource-name>)
                    n225 = Concatenate Strings("SLVL " ("chaîne"), w351) -> (w349:string)
                    n226 = VISA Write(VISA resource name=w347, write buffer=w349) -> ()  [unwired: 1 in, 3 out]
                  }
                }
              }
              frame "Fixarray" {
                n227 = local read "Fix Instrument"() -> (w353:string)
                n228 = local read "Conversion Factor Fix\n1 V = ??"() -> (w356:dbl)
                n229 = Divide(x=w355, y=w356) -> (x/y=w354:dbl)
                n230 = case shown="\"DAC\"" w353 {
                  tunnel: w354 -> [_ w358 w361 w363 w365]
                  frame Default {
                  }
                  frame "DAC" {
                    n231 = local read "DAC 2 number"() -> (w357:u8)
                    n232 = call "SetDAC_04.vi"("RS232/ Optical Fiber"=refnum<visa-resource-name> "COM1", "DATA (V)"=w358, "DAC nr"=w357) -> ()  [unwired: 2 in, 1 out]
                  }
                  frame "K2400_2" {
                    n233 = local read "K2400 2"() -> (w360:refnum<visa-resource-name>)
                    n234 = call "K2400_ApplyVOLTsafe_GUMS.vi"("Voltage target [V]"=w361, "VISA Resource Name"=w360) -> ()  [unwired: 1 out]
                  }
                  frame "K2400_1" {
                    n235 = local read "K2400 1"() -> (w362:refnum<visa-resource-name>)
                    n236 = call "K2400_ApplyVOLTsafe_GUMS.vi"("Voltage target [V]"=w363, "VISA Resource Name"=w362) -> ()  [unwired: 1 out]
                  }
                  frame "Lockin" {
                    n237 = Number To Fractional String(number=w365) -> (F-format string=w368:string)  [unwired: 3 out]
                    n238 = local read "Lockin1"() -> (w364:refnum<visa-resource-name>)
                    n239 = Concatenate Strings("SLVL " ("chaîne"), w368) -> (w366:string)
                    n240 = VISA Write(VISA resource name=w364, write buffer=w366) -> ()  [unwired: 1 in, 3 out]
                  }
                }
              }
              frame Default {
              }
              frame "Bfield" {
                n241 = node(w370) -> (w369:dbl[unit])
                n242 = local read "Sweep Rate [T/min]"() -> (w371:dbl)
                n243 = node(w371) -> (w372:dbl[unit])
                n244 = call "TeslSetField.vi"("Sweep rate"=w372, "Field required:"=w369) -> ()  [unwired: 2 in, 2 out]
              }
              frame "Temperature" {
                n245 = local read "ITC ref"() -> (w373:T2)
                n246 = call "Tloop.vi"("ITCSignal"=w373, "Regulate ?"=TRUE) -> ()  [unwired: 3 in, 2 out]
              }
            }
            n247 = for {
              N: w340 -> [w381]
              tunnel: w339 -> [w398]
              tunnel: w338 -> [w395]
              tunnel: w334 -> [w393]
              tunnel: w333 -> [w392]
              tunnel: w332 -> [_]
              tunnel: w325 -> [w380]
              tunnel: w324 -> [w384]
              tunnel: [w376] -> w323
              i -> [w382]
              stop <- w376 stop-if-true
              n248 = Multiply(x=w381, y=w380) -> (x*y=w378:i32)
              n249 = global write "stopButton.vi" "stopsignal"(FALSE) -> ()
              n250 = Multiply(x=w381, y=w382) -> (x*y=w379:i32)
              n251 = Add(x=w382, y=w380) -> (x+y=w385:i32)
              n252 = Increment(x=w382) -> (x+1=w386:i32)
              n253 = local read "Device Cluster"() -> (w388:T4)
              n254 = local read "Gain Cluster 2"() -> (w387:T1)
              n255 = Add(x=w379, y=w378) -> (x+y=w377:i32)
              n256 = call "autoNameFile.vi"("num"=w385, "File Basename"="File Basename", "Folder Name"="Folder Name") -> ("path"=w401:path)
              n257 = Index Array(array=w395, index (row)=w386, index (col)=1 ("disabled index (col)")) -> (element=w394:dbl)
              n258 = case shown="\"Bfield\"" w393 {
                selector: w393 -> [_ _ w436 _ _]
                tunnel: w394 -> [w405 w424 _ w440 _]
                tunnel: TRUE ("SaveDataQuery") -> [w402 w421 w437 w438 w445]
                tunnel: [w402 w421 w437 w438 w445] -> w390
                tunnel: [_ _ w436 _ _] -> w389
                frame "sweeparray" {
                  n259 = local read "Sweep Instrument"() -> (w403:string)
                  n260 = local read "Conversion Factor Sweep\n1 V = ??"() -> (w406:dbl)
                  n261 = Divide(x=w405, y=w406) -> (x/y=w404:dbl)
                  n262 = case shown="\"DAC\"" w403 {
                    tunnel: w404 -> [_ w409 w413 w415 w417]
                    frame Default {
                    }
                    frame "DAC" {
                      n263 = Multiply(x=w409, y=1000.0) -> (x*y=w411:dbl)
                      n264 = local read "DAC 1 number"() -> (w407:u8)
                      n265 = local read "DAC"() -> (w408:refnum<visa-resource-name>)
                      n266 = call "DAC set.vi"("DAC number"=w407, "DAC set [mV]"=w411, "DAC COM port"=w408) -> ()  [unwired: 1 out]
                    }
                    frame "K2400_2" {
                      n267 = local read "K2400 2"() -> (w412:refnum<visa-resource-name>)
                      n268 = call "K2400_ApplyVOLTsafe_GUMS.vi"("Voltage target [V]"=w413, "VISA Resource Name"=w412) -> ()  [unwired: 1 out]
                    }
                    frame "K2400_1" {
                      n269 = local read "K2400 1"() -> (w414:refnum<visa-resource-name>)
                      n270 = call "K2400_ApplyVOLTsafe_GUMS.vi"("Voltage target [V]"=w415, "VISA Resource Name"=w414) -> ()  [unwired: 1 out]
                    }
                    frame "Lockin" {
                      n271 = Number To Fractional String(number=w417) -> (F-format string=w420:string)  [unwired: 3 out]
                      n272 = local read "Lockin1"() -> (w416:refnum<visa-resource-name>)
                      n273 = Concatenate Strings("SLVL " ("chaîne"), w420) -> (w418:string)
                      n274 = VISA Write(VISA resource name=w416, write buffer=w418) -> ()  [unwired: 1 in, 3 out]
                    }
                  }
                }
                frame "Fixarray" {
                  n275 = local read "Fix Instrument"() -> (w422:string)
                  n276 = local read "Conversion Factor Fix\n1 V = ??"() -> (w425:dbl)
                  n277 = Divide(x=w424, y=w425) -> (x/y=w423:dbl)
                  n278 = case shown="\"DAC\"" w422 {
                    tunnel: w423 -> [_ w427 w429 w430 w432]
                    frame Default {
                    }
                    frame "DAC" {
                      n279 = local read "DAC 2 number"() -> (w426:u8)
                      n280 = call "SetDAC_04.vi"("RS232/ Optical Fiber"=refnum<visa-resource-name> "COM1", "DATA (V)"=w427, "DAC nr"=w426) -> ()  [unwired: 2 in, 1 out]
                    }
                    frame "K2400_2" {
                      n281 = call "K2400_ApplyVOLTsafe_GUMS.vi"("Voltage target [V]"=w429) -> ()  [unwired: 1 in, 1 out]
                    }
                    frame "K2400_1" {
                      n282 = call "K2400_ApplyVOLTsafe_GUMS.vi"("Voltage target [V]"=w430) -> ()  [unwired: 1 in, 1 out]
                    }
                    frame "Lockin" {
                      n283 = Number To Fractional String(number=w432) -> (F-format string=w435:string)  [unwired: 3 out]
                      n284 = local read "Lockin1"() -> (w431:refnum<visa-resource-name>)
                      n285 = Concatenate Strings("SLVL " ("chaîne"), w435) -> (w433:string)
                      n286 = VISA Write(VISA resource name=w431, write buffer=w433) -> ()  [unwired: 1 in, 3 out]
                    }
                  }
                }
                frame Default {
                }
                frame "Bfield" {
                  n287 = node(w440) -> (w439:dbl[unit])
                  n288 = local read "Sweep Rate [T/min]"() -> (w441:dbl)
                  n289 = node(w441) -> (w442:dbl[unit])
                  n290 = call "TeslSetField.vi"("Sweep rate"=w442, "Field required:"=w439) -> ()  [unwired: 2 in, 2 out]
                }
                frame "Temperature" {
                  n291 = local read "ITC ref"() -> (w443:T2)
                  n292 = call "Tloop.vi"("ITCSignal"=w443, "Regulate ?"=TRUE) -> ()  [unwired: 3 in, 2 out]
                }
              }
              n293 = for {
                N: w398 -> [_]
                tunnel: [TRUE ("stopsignal")] -> w397
                tunnel: w395 -> [w458]
                tunnel: w392 -> [w456]
                tunnel: w389 -> [_]
                tunnel: w384 -> [w454]
                tunnel: w377 -> [w451]
                tunnel: [w449] -> w376
                i -> [w452]
                stop <- w449 stop-if-true
                n294 = local read "Cancel run"() -> (w449:bool)
                n295 = Add(x=w452, y=w451) -> (x+y=w450:i32)
                n296 = Increment(x=w452) -> (x+1=w455:i32)
                n297 = local read "Step Delay (ms)"() -> (w447:dbl)
                n298 = Divide(x=w450, y=w454) -> (x/y=→"Total Progress":dbl)
                n299 = Index Array(array=w458, index (row)=w455, index (col)=0 ("disabled index (col)")) -> (element=w448:dbl)
                n300 = local write "Current sweep"(w448) -> ()
                n301 = Wait (ms)(milliseconds to wait=w447) -> (millisecond timer value=w446:u32)
                n302 = case shown="\"Bfield\"" w456 {
                  tunnel: w448 -> [w462 w480 _ w495 w499]
                  tunnel: w446 -> [_ _ _ _ _]
                  frame "sweeparray" {
                    n303 = local read "Sweep Instrument"() -> (w460:string)
                    n304 = local read "Conversion Factor Sweep\n1 V = ??"() -> (w463:dbl)
                    n305 = Divide(x=w462, y=w463) -> (x/y=w461:dbl)
                    n306 = case shown="\"DAC\"" w460 {
                      tunnel: w461 -> [_ w466 w468 w471 w474]
                      tunnel: [_ _ _ w469 w472] -> _
                      frame Default {
                      }
                      frame "DAC" {
                        n307 = local read "DAC 1 number"() -> (w465:u8)
                        n308 = call "SetDAC_04.vi"("RS232/ Optical Fiber"=refnum<visa-resource-name> "COM1", "DATA (V)"=w466, "DAC nr"=w465) -> ()  [unwired: 2 in, 1 out]
                      }
                      frame "K2400_2" {
                        n309 = local read "K2400 2"() -> (w467:refnum<visa-resource-name>)
                        n310 = call "K2400setV.vi"("Voltage target [V]"=w468, "VISA Resource Name"=w467) -> ()  [unwired: 1 in, 2 out]
                      }
                      frame "K2400_1" {
                        n311 = local read "K2400 1"() -> (w470:refnum<visa-resource-name>)
                        n312 = call "K2400setV.vi"("Voltage target [V]"=w471, "VISA Resource Name"=w470) -> ("error out"=w469:errorcluster)  [unwired: 1 in, 1 out]
                      }
                      frame "Lockin" {
                        n313 = Number To Fractional String(number=w474) -> (F-format string=w477:string)  [unwired: 3 out]
                        n314 = local read "Lockin1"() -> (w473:refnum<visa-resource-name>)
                        n315 = Concatenate Strings("SLVL " ("chaîne"), w477) -> (w475:string)
                        n316 = VISA Write(VISA resource name=w473, write buffer=w475) -> (error out=w472:errorcluster)  [unwired: 1 in, 2 out]
                      }
                    }
                  }
                  frame "Fixarray" {
                    n317 = local read "Fix Instrument"() -> (w478:string)
                    n318 = local read "Conversion Factor Fix\n1 V = ??"() -> (w481:dbl)
                    n319 = Divide(x=w480, y=w481) -> (x/y=w479:dbl)
                    n320 = case shown="\"DAC\"" w478 {
                      tunnel: w479 -> [_ w483 w486 w488 w490]
                      frame Default {
                      }
                      frame "DAC" {
                        n321 = local read "DAC 1 number"() -> (w482:u8)
                        n322 = call "SetDAC_04.vi"("RS232/ Optical Fiber"=refnum<visa-resource-name> "COM1", "DATA (V)"=w483, "DAC nr"=w482) -> ()  [unwired: 2 in, 1 out]
                      }
                      frame "K2400_2" {
                        n323 = local read "K2400 2"() -> (w485:refnum<visa-resource-name>)
                        n324 = call "K2400_ApplyVOLTsafe_GUMS.vi"("Voltage target [V]"=w486, "VISA Resource Name"=w485) -> ()  [unwired: 1 out]
                      }
                      frame "K2400_1" {
                        n325 = local read "K2400 1"() -> (w487:refnum<visa-resource-name>)
                        n326 = call "K2400_ApplyVOLTsafe_GUMS.vi"("Voltage target [V]"=w488, "VISA Resource Name"=w487) -> ()  [unwired: 1 out]
                      }
                      frame "Lockin" {
                        n327 = Number To Fractional String(number=w490) -> (F-format string=w493:string)  [unwired: 3 out]
                        n328 = local read "Lockin1"() -> (w489:refnum<visa-resource-name>)
                        n329 = Concatenate Strings("SLVL " ("chaîne"), w493) -> (w491:string)
                        n330 = VISA Write(VISA resource name=w489, write buffer=w491) -> ()  [unwired: 1 in, 3 out]
                      }
                    }
                  }
                  frame Default {
                  }
                  frame "Bfield" {
                    n331 = node(w495) -> (w494:dbl[unit])
                    n332 = local read "Sweep Rate [T/min]"() -> (w496:dbl)
                    n333 = node(w496) -> (w497:dbl[unit])
                    n334 = call "TeslSetField.vi"("Sweep rate"=w497, "Field required:"=w494) -> ()  [unwired: 2 in, 2 out]
                  }
                  frame "Temperature" {
                    n335 = local read "ITC ref"() -> (w500:T2)
                    n336 = call "Tloop.vi"("ITCSignal"=w500, "T target [K]"=w499, "Regulate ?"=TRUE) -> ()  [unwired: 2 in, 2 out]
                  }
                }
              }
              n337 = call "gums_measureLoop.vi"("File Name"=w401, "SaveDataQuery"=w390, "Gain Cluster 2"=w387, "Refresh Rate [ms]"="Refresh Rate [ms]", "Device Cluster"=w388) -> ()  [unwired: 6 in]
              n338 = global write "stopButton.vi" "stopsignal"(w397) -> ()
            }
          }
        }
        n339 = local write "START"(w241) -> ()
      }
      frame "mainLoop" {
        n340 = global write "stopButton.vi" "stopsignal"(FALSE) -> ()
        n341 = local read "Sweep back\nto zero?"() -> (w513:bool)
        n342 = local read "Sweep Rate [T/min]"() -> (w507:dbl)
        n343 = local read "Priority type array"() -> (w532:string[])
        n344 = local read "Device Cluster"() -> (w526:T4)
        n345 = local read "Gain Cluster 2"() -> (w534:T1)
        n346 = global read "GlobalVar.vi" "LaserControl"() -> (w502:T7)
        n347 = local read "Loop Cluster"() -> (w535:T6)
        n348 = global write "GlobalVar.vi" "Set Persistent"("Set Persistent") -> ()
        n349 = local read "Total sweep sequence"() -> (w536:dbl[][])
        n350 = Bundle By Name(cluster=w502, "Power Stabilization"="Power stabilization") -> (w504:T7)
        n351 = global write "GlobalVar.vi" "Sweep rate [T/min]"(w507) -> ()
        n352 = local read "Conversion Factor Sweep\n1 V = ??"() -> (w528:dbl)
        n353 = local read "Conversion Factor Fix\n1 V = ??"() -> (w527:dbl)
        n354 = global write "GlobalVar.vi" "LaserControl"(w504) -> ()
        n355 = Index Array(array=w536, index (row)=0) -> (element=w519:dbl[])  [unwired: 1 in]
        "Num elements in col" <- w519
        n356 = Array Size(array=w519) -> (size(s)=w521:i32)
        n357 = Array Size(array=w519) -> (size(s)=w541:i32)
        n358 = Array Subset(array=w519, index=1) -> (w539:dbl[])  [unwired: 1 in]
        n359 = Unbundle By Name(w535) -> ("Sweep Instrument"=w529:string, "Fix Instrument"=w501:string, "Wavelength"=w503:bool)  [unwired: 6 out]
        n360 = Array Size(array=w539) -> (size(s)=w543:i32)
        n361 = Unbundle By Name(w526) -> ("K2400 1"=w525:refnum<visa-resource-name>, "K2400 2"=w524:refnum<visa-resource-name>, "Lockin1"=w523:refnum<visa-resource-name>, "ITC signal"=w522:T2)
        n362 = Decrement(x=w521) -> (x-1=w520:i32)
        n363 = Initialize Array(1, w541) -> (→"row state":i32[])
        n364 = for {
          N: w520 -> [_]
          tunnel: w519 -> [w564]
          shift-right: [w561] -> w517
          shift-left: 1 ("index") -> [w562]
          i -> [w566]
          n365 = Increment(x=w566) -> (x+1=w565:i32)
          n366 = Index Array(array=w564, index=w565) -> (element=w563:dbl)
          n367 = Multiply(x=w562, y=w563) -> (x*y=w561:dbl)
        }
        "TotalPnts" <- w517
        n368 = while {
          tunnel: w543 -> [_]
          shift-right: [w592] -> _
          shift-left: "start" -> [w593]
          tunnel: w536 -> [w591]
          tunnel: w534 -> [w590]
          tunnel: w526 -> [w589]
          tunnel: w532 -> [w588]
          tunnel: [w572] -> w531
          tunnel: "init" -> [w587]
          tunnel: [w587] -> w515
          tunnel: w501 -> [w586]
          tunnel: w529 -> [w585]
          tunnel: w507 -> [w584]
          tunnel: w507 -> [w583]
          tunnel: w507 -> [w582]
          tunnel: w528 -> [w581]
          tunnel: w527 -> [w580]
          tunnel: w525 -> [w579]
          tunnel: w524 -> [w578]
          tunnel: w523 -> [w577]
          tunnel: w522 -> [w576]
          tunnel: [w571] -> w510
          tunnel: [w570] -> w509
          tunnel: [w569] -> w508
          tunnel: w503 -> [w568]
          tunnel: w502 -> [w567]
          stop <- w572 stop-if-true
          n369 = case shown="\"sweep\"" w593 {
            selector: w593 -> [_ _ _ w788]
            tunnel: ["sweep" w683 w740 w788] -> w592
            tunnel: w591 -> [w610 w685 w736 _]
            tunnel: [_ _ _ TRUE] -> w574
            tunnel: w590 -> [_ w677 _ _]
            tunnel: w589 -> [_ w676 _ _]
            tunnel: w588 -> [w609 w671 w735 _]
            tunnel: w586 -> [w607 w668 w734 _]
            tunnel: w585 -> [w608 w667 w733 _]
            tunnel: w584 -> [_ _ w732 _]
            tunnel: w583 -> [w606 _ _ _]
            tunnel: w582 -> [_ w666 _ _]
            tunnel: w581 -> [w605 w665 w730 _]
            tunnel: w580 -> [w604 w664 w731 _]
            tunnel: w579 -> [w601 w663 w726 _]
            tunnel: w578 -> [w602 w662 w727 _]
            tunnel: w577 -> [w600 w661 w728 _]
            tunnel: w576 -> [w603 w660 w729 _]
            tunnel: FALSE ("stopsignal") -> [_ w659 _ _]
            tunnel: [_ w655 _ _] -> w573
            tunnel: [_ w647 _ _] -> w571
            tunnel: [_ w646 _ _] -> w570
            tunnel: [_ w645 _ _] -> w569
            tunnel: w568 -> [w598 _ _ _]
            tunnel: w567 -> [w594 _ _ _]
            frame "start", Default {
              n370 = local read "row state"() -> (w613:i32[])
              n371 = local read "Power stabilization"() -> (w597:bool)
              n372 = And(x=w598, y=w597) -> (x .and. y?=w596:bool)
              n373 = case shown="True" w596 {
                tunnel: [_ w618] -> w595
                tunnel: w594 -> [_ w615]
                frame False {
                }
                frame True {
                  n374 = global read "perHandlemonochromator.vi" "peHandle"() -> (w622:u32)
                  n375 = call "PE Get Wavelength.vi"("peHandle"=w622) -> ("error out"=w619:errorcluster, "wavelength"=w621:dbl)  [unwired: 8 in, 1 out]
                  n376 = call "GetPower.vi"("error in (no error)"=w619, "Wavelength (nm)"=w621, "Input Device"=refnum<visa-resource-name> "USB0::0x1313::0x8072::P2007928::INSTR") -> ("error out"=w618:errorcluster, "Power (W)"=w617:dbl)  [unwired: 1 in, 2 out]
                  n377 = Bundle By Name(cluster=w615, "Laser Power [W]"=w617) -> (w616:T7)
                  n378 = local write "Laser Power [W]"(w617) -> ()
                  n379 = global write "GlobalVar.vi" "LaserControl"(w616) -> ()
                }
              }
              n380 = Array Size(array=w613) -> (size(s)=w612:i32)
              n381 = for {
                N: w612 -> [w640]
                tunnel: 1 -> [w641]
                tunnel: w610 -> [w642]
                tunnel: w609 -> [w636]
                tunnel: w608 -> [w634]
                tunnel: w607 -> [w633]
                tunnel: w606 -> [_]
                tunnel: w605 -> [w632]
                tunnel: w604 -> [w631]
                tunnel: w603 -> [w630]
                tunnel: w602 -> [w629]
                tunnel: w601 -> [w628]
                tunnel: w600 -> [w627]
                tunnel: [w626] -> _
                tunnel: [0 ("Current col")] -> w599
                tunnel: w595 -> [_]
                i -> [w639]
                n382 = Increment(x=w639) -> (x+1=w638:i32)
                n383 = Subtract(x=w640, y=w638) -> (x-y=w635:i32)
                n384 = Index Array(array=w636, index=w635) -> (element=w623:string)
                n385 = Index Array(array=w642, index (row)=w641, index (col)=w635) -> (element=w637:dbl)
                n386 = case shown="\"Fixarray\"" w623 {
                  tunnel: [w643 w644] -> w624
                  frame "Fixarray" {
                    n387 = local read "DAC 2 number"() -> (w643:u8)
                  }
                  frame "sweeparray", Default {
                    n388 = local read "DAC 1 number"() -> (w644:u8)
                  }
                }
                n389 = call "ApplyInstrument.vi"("Instrument"=w623, "ITC ref"=w630, "Conversion Factor Fix\n1 V = ??"=w631, "K2400 1"=w628, "Sweep Instrument"=w634, "Valin"=w637, "Fix Instrument"=w633, "DAC number"=w624, "K2400 2"=w629, "Conversion Factor Sweep\n1 V = ??"=w632, "Lockin1"=w627) -> ("error out"=w626:errorcluster)  [unwired: 4 in]
              }
              n390 = local write "Current col"(w599) -> ()
            }
            frame "sweep" {
              w689 = 0 ("index")
              n391 = global write "stopButton.vi" "stopsignal"(w659) -> ()
              n392 = Index Array(array=w685, index (row)=w689, index (col)=w689) -> (element=w688:dbl)
              n393 = local read "Current col"() -> (w669:i32)
              n394 = local read "TotalPnts"() -> (w658:dbl)
              n395 = local read "row state"() -> (w682:i32[])
              n396 = local read "counter"() -> (w650:i32)
              n397 = local read "Refresh Rate [ms]"() -> (w656:i32)
              n398 = local read "Sweep Toothsaw"() -> (w648:bool)
              n399 = local read "File Basename"() -> (w674:string)
              n400 = local read "Folder Name"() -> (w675:path)
              n401 = Index Array(array=w671, index=w669) -> (element=w670:string)
              n402 = Increment(x=w650) -> (x+1=w654:i32)
              n403 = Quotient & Remainder(x=w650, y=2.0) -> (x-y*floor(x/y)=w652:dbl)  [unwired: 1 out]
              n404 = local write "counter"(w654) -> ()
              n405 = Index Array(array=w682, index=w669) -> (element=w686:i32)
              n406 = call "autoNameFile.vi"("num"=w650, "File Basename"=w674, "Folder Name"=w675) -> ("path"=w678:path)
              n407 = Not Equal To 0?(x=w652) -> (x != 0?=w649:bool)
              n408 = for {
                N: w688 -> [_]
                tunnel: [w715] -> w683
                tunnel: "changerow" -> [w715]
                tunnel: w669 -> [w703]
                tunnel: w685 -> [w704]
                tunnel: [w703] -> w680
                shift-right: [w714] -> _
                shift-left: w686 -> [w702]
                tunnel: [TRUE] -> w673
                tunnel: w670 -> [w697]
                tunnel: [w691] -> _
                tunnel: w668 -> [w693]
                tunnel: w667 -> [w711]
                tunnel: w666 -> [_]
                tunnel: w665 -> [w710]
                tunnel: w664 -> [w709]
                tunnel: w663 -> [w695]
                tunnel: w662 -> [w694]
                tunnel: w661 -> [w708]
                tunnel: w660 -> [w707]
                tunnel: [w706] -> w655
                tunnel: [w705] -> _
                tunnel: w654 -> [w705]
                tunnel: [w705] -> w653
                tunnel: w649 -> [w701]
                tunnel: w648 -> [w698]
                tunnel: [w695] -> w647
                tunnel: [w694] -> w646
                tunnel: [w693] -> w645
                stop <- w706 stop-if-true
                n409 = case shown="\"Fixarray\"" w697 {
                  tunnel: [w716 w717] -> w696
                  frame "Fixarray" {
                    n410 = local read "DAC 2 number"() -> (w716:u8)
                  }
                  frame "sweeparray", Default {
                    n411 = local read "DAC 1 number"() -> (w717:u8)
                  }
                }
                n412 = And(x=w701, y=w698) -> (x .and. y?=w700:bool)
                n413 = Increment(x=w702) -> (x+1=w714:i32)
                n414 = local read "Cancel run"() -> (w706:bool)
                n415 = local read "Step Delay (ms)"() -> (w690:dbl)
                n416 = case shown="False" w700 {
                  tunnel: w702 -> [w718 w721]
                  tunnel: w704 -> [_ w725]
                  tunnel: w703 -> [_ w723]
                  tunnel: [w718 w720] -> w699
                  frame False {
                    # "forth"
                  }
                  frame True {
                    n417 = Decrement(x=w721) -> (x-1=w719:i32)
                    n418 = Index Array(array=w725, index (row)=0, index (col)=w723) -> (element=w722:dbl)
                    n419 = Subtract(x=w722, y=w719) -> (x-y=w720:dbl)
                  }
                }
                n420 = Index Array(array=w704, index (row)=w699, index (col)=w703) -> (element=w712:dbl)
                n421 = call "ApplyInstrument.vi"("Instrument"=w697, "ITC ref"=w707, "Conversion Factor Fix\n1 V = ??"=w709, "K2400 1"=w695, "Sweep Instrument"=w711, "Valin"=w712, "Fix Instrument"=w693, "DAC number"=w696, "K2400 2"=w694, "Conversion Factor Sweep\n1 V = ??"=w710, "Lockin1"=w708) -> ("error out"=w692:errorcluster)  [unwired: 4 in]
                n422 = call "wait.vi"("error in (no error)"=w692, "wait time"=w690) -> ("error in (no error) 2"=w691:errorcluster)
              }
              n423 = call "gums_measureLoop.vi"("File Name"=w678, "SaveDataQuery"=TRUE, "Gain Cluster 2"=w677, "Refresh Rate [ms]"=w656, "Device Cluster"=w676) -> ()  [unwired: 6 in]
              n424 = global write "stopButton.vi" "stopsignal"(w673) -> ()
              n425 = Divide(x=w653, y=w658) -> (x/y=w657:dbl)
              n426 = Increment(x=w680) -> (x+1=w684:i32)
              n427 = Replace Array Subset(array=w682, new element=1 ("new element/subarray"), index=w680) -> (w681:i32[])
              n428 = local write "Current col"(w684) -> ()
              n429 = local write "row state"(w681) -> ()
              n430 = local write "Total Progress"(w657) -> ()
            }
            frame "changerow" {
              n431 = local read "Current col"() -> (w737:i32)
              n432 = local read "row state"() -> (w747:i32[])
              n433 = local read "Num elements in col"() -> (w745:i32[])
              n434 = Index Array(array=w747, index=w737) -> (element=w743:i32)
              n435 = Increment(x=w743) -> (x+1=w742:i32)
              n436 = Index Array(array=w745, index=w737) -> (element=w750:i32)
              n437 = Array Size(array=w745) -> (size(s)=w744:i32)
              n438 = Greater?(x=w742, y=w750) -> (0:w749:bool)
              n439 = case shown="False" w749 {
                tunnel: [w776 0] -> w738
                tunnel: w742 -> [w776 _]
                tunnel: [w774 w782] -> w748
                tunnel: [w771 w779] -> w741
                tunnel: w737 -> [w775 w783]
                tunnel: w744 -> [_ w781]
                frame False {
                  n440 = Decrement(x=w775) -> (x-1=w774:i32)
                  n441 = Equal?(x=0, y=w774) -> (x = y?=w772:bool)
                  n442 = case shown="False" w772 {
                    tunnel: ["changerow" "sweep"] -> w771
                    frame False {
                    }
                    frame True {
                    }
                  }
                }
                frame True {
                  n443 = Increment(x=w783) -> (x+1=w782:i32)
                  n444 = Greater?(x=w782, y=w781) -> (0:w780:bool)
                  n445 = case shown="False" w780 {
                    tunnel: ["changerow" "stop"] -> w779
                    frame False {
                    }
                    frame True {
                    }
                  }
                }
              }
              n446 = local write "Current col"(w748) -> ()
              n447 = Replace Array Subset(array=w747, new element=w738, index=w737) -> (w746:i32[])
              n448 = Not Equal To 0?(x=w738) -> (x != 0?=w739:bool)
              n449 = local write "row state"(w746) -> ()
              n450 = case shown="True" w739 {
                tunnel: w741 -> [w751 w768]
                tunnel: [w751 w768] -> w740
                tunnel: w736 -> [_ w767]
                tunnel: w737 -> [_ w762]
                tunnel: w738 -> [_ w766]
                tunnel: w735 -> [_ w763]
                tunnel: w734 -> [_ w761]
                tunnel: w733 -> [_ w760]
                tunnel: w732 -> [_ _]
                tunnel: w731 -> [_ w759]
                tunnel: w730 -> [_ w758]
                tunnel: w729 -> [_ w757]
                tunnel: w728 -> [_ w756]
                tunnel: w727 -> [_ w755]
                tunnel: w726 -> [_ w754]
                frame False {
                }
                frame True {
                  n451 = Index Array(array=w767, index (row)=w766, index (col)=w762) -> (element=w764:dbl)
                  n452 = Index Array(array=w763, index=w762) -> (element=w753:string)
                  n453 = Wait (ms)(milliseconds to wait=u32 400) -> ()  [unwired: 1 out]
                  n454 = case shown="\"Fixarray\"" w753 {
                    tunnel: [w769 w770] -> w752
                    frame "Fixarray" {
                      n455 = local read "DAC 2 number"() -> (w769:u8)
                    }
                    frame "sweeparray", Default {
                      n456 = local read "DAC 1 number"() -> (w770:u8)
                    }
                  }
                  n457 = call "ApplyInstrument.vi"("Instrument"=w753, "ITC ref"=w757, "Conversion Factor Fix\n1 V = ??"=w759, "K2400 1"=w754, "Sweep Instrument"=w760, "Valin"=w764, "Fix Instrument"=w761, "DAC number"=w752, "K2400 2"=w755, "Conversion Factor Sweep\n1 V = ??"=w758, "Lockin1"=w756) -> ()  [unwired: 4 in, 1 out]
                }
              }
            }
            frame "stop" {
            }
          }
          n458 = Or(x=w574, y=w573) -> (x .or. y?=w572:bool)
        }
        n459 = Not(x=w531) -> (.not. x?=w514:bool)
        n460 = case shown="True" "Sweep Field back to zero" {
          tunnel: w515 -> [w555 w560]
          tunnel: [w555 w560] -> w512
          frame False {
          }
          frame True {
            n461 = node("Zero ramp Rate [T/min] 2") -> (w559:dbl[unit])
            n462 = node(0.0) -> (w558:dbl[unit])
            n463 = call "TeslSetField.vi"("Sweep rate"=w559, "Field required:"=w558) -> ()  [unwired: 2 in, 2 out]
          }
        }
        n464 = local write "START"(w514) -> ()
        n465 = global write "stopButton.vi" "stopsignal"(w514) -> ()
        n466 = case shown="True" w513 {
          tunnel: w512 -> [w547 w554]
          tunnel: [w547 w554] -> w511
          tunnel: w510 -> [_ w550]
          tunnel: w509 -> [_ w549]
          tunnel: w508 -> [_ _]
          tunnel: w501 -> [_ w548]
          frame False {
          }
          frame True {
            n467 = local read "DAC 2 number"() -> (w551:u8)
            n468 = call "ApplyInstrument.vi"("Instrument"="Fixarray", "K2400 1"=w550, "Valin"=0.0, "Fix Instrument"=w548, "DAC number"=w551, "K2400 2"=w549) -> ()  [unwired: 9 in, 1 out]
          }
        }
        "Current col" <- -1 ("Current col")
        "counter" <- 0 ("counter")
      }
      frame "loopIncrease" {
        w801 = 1 ("Nb Sweep Indicator")
        n469 = local read "Nb steps 2"() -> (w796:i32)
        n470 = local read "Nb steps"() -> (w795:i32)
        n471 = local write "Priority B"(w801) -> ()
        n472 = local write "Nb Sweep Indicator"(w801) -> ()
        n473 = local read "Nb Loop Indicator"() -> (w804:i32)
        n474 = local read "sweep stop 2 [V]"() -> (w797:dbl)
        n475 = local read "sweep stop [V]"() -> (w799:dbl)
        n476 = Add(x="Nb steps Increase 2", y=w796) -> (x+y=w792:dbl)
        n477 = Add(x=w797, y="Gate Increase 2 (V)") -> (x+y=w789:dbl)
        n478 = Add(x="Gate Increase (V)", y=w799) -> (x+y=w790:dbl)
        n479 = Add(x="Nb steps Increase", y=w795) -> (x+y=w791:dbl)
        n480 = Increment(x=w804) -> (x+1=w803:i32)
        n481 = local write "Nb steps 2"(w792) -> ()
        n482 = local write "sweep stop 2 [V]"(w789) -> ()
        n483 = local write "sweep stop [V]"(w790) -> ()
        n484 = local write "Nb steps"(w791) -> ()
        n485 = local write "Nb Loop Indicator"(w803) -> ()
      }
      frame "endRun" {
        n486 = local read "Device Cluster"() -> (w806:T4)
        n487 = case shown="True" "Sweep back to zero" {
          frame False {
          }
          frame True {
            n488 = call "K2400_ApplyVOLTsafe_GUMS.vi"("Voltage target [V]"=0.0) -> ()  [unwired: 2 in]
          }
        }
        n489 = Unbundle By Name(w806) -> ("DAC present"=w805:bool)
        n490 = case shown="True" w805 {
          frame False {
          }
          frame True {
            n491 = local read "DAC"() -> (w810:refnum<visa-resource-name>)
            n492 = call "closeRS232.vi"("VISA resource name"=w810) -> ()  [unwired: 2 in]
          }
        }
      }
      frame "EmptyArrays" {
        w813 = 0.0
        n493 = Initialize Array(w813, w813) -> (w812:dbl[])
        n494 = local write "B [T]"(w812) -> ()
        n495 = local write "T [K]"(w812) -> ()
        n496 = local write "Sweep Bias"(w812) -> ()
        n497 = local write "Fix Bias"(w812) -> ()
      }
      frame "DACioload" {
        n498 = local read "DACindic"() -> (w817:bool)
        n499 = local read "DAC"() -> (w818:refnum<visa-resource-name>)
        n500 = case shown="False" w817 {
          tunnel: w818 -> [w820 w822]
          tunnel: "init" -> [w819 w821]
          tunnel: [w819 w821] -> w815
          frame False {
            n501 = call "closeRS232.vi"("VISA resource name"=w820) -> ()  [unwired: 2 in]
          }
          frame True {
            n502 = call "openRS232.vi"("com"=w822) -> ("VISA resource name"=w823:refnum<visa-resource-name>)  [unwired: 1 out]
            n503 = global write "Visa name1.vi" "VISA name"(w823) -> ()
          }
        }
      }
    }
    "x .or. y?" <- w28
  }
  n504 = Unbundle By Name("Gain Cluster 2") -> ("conversion factor BG"=→"conversion factor sweep":dbl, "Vin / Vout 1"=→"Bias factor":dbl)  [unwired: 10 out]
  n505 = Unbundle By Name("Device Cluster") -> ("K2400 1"=→"K2400 1":refnum<visa-resource-name>, "Lockin1"=→"Lockin1":refnum<visa-resource-name>, "K2400 2"=→"K2400 2":refnum<visa-resource-name>, "DAC"=w2:refnum<visa-resource-name>, "DAC sweep"=→"DAC 1 number":u8, "ITC signal"=→"ITC ref":T2, "DAC fix"=→"DAC 2 number":u8, "DAC present"=w3:bool)  [unwired: 1 out]
  "DAC" <- w2
  n506 = case shown="True" w3 {
    tunnel: w2 -> [_ w824]
    frame False {
    }
    frame True {
      n507 = call "openRS232.vi"("com"=w824) -> ("VISA resource name"=w825:refnum<visa-resource-name>)  [unwired: 1 out]
      n508 = global write "Visa name1.vi" "VISA name"(w825) -> ()
    }
  }
  "Nb Sweep Indicator" <- 1 ("Nb Sweep Indicator")
  "Nb Loop Indicator" <- 0.0 ("Nb Sweep Indicator")
